vi "r3_Pick&Place_module_sensor.vi"() -> ()   [LabVIEW 2016]
uses:
  Classes/Controllers/I-O/Copy of NI-DAQ Folder/NI-DAQ.lvclass
  D:/INTT/V1/Classes/Controllers/I-O/Copy of I-O Folder/I-O.lvclass
  Classes/Controllers/Dispenser/Copy of Ultimus V2 Folder/Ultimus V2.lvclass
  <vilib>/Analysis/coordinate.llb/2D Cartesian Coordinate Rotation (Scalar).vi
  <vilib>/Utility/file.llb/Read Delimited Spreadsheet (DBL).vi
  <vilib>/Utility/file.llb/Write Delimited Spreadsheet (DBL).vi
  Classes/Controllers/Motion/Copy of Motion Folder/Motion.lvclass
  Classes/Controllers/Camera/Copy of Controller Folder/Controller.lvclass
  <vilib>/Analysis/NI_AALPro.lvlib
  Classes/Controllers/I-O/Copy of I-O Folder/I-O.lvclass
panel:
  in  "sensor pad offset":dbl[][](array[numeric])=[[0.01279, -0.02707, 0.0, 0.0], [0.00738, -0.02377, 0.0, 0.0]]
  out "Sample on HDI aspect to drawing":dbl[][](array[numeric]) format="%#_8g"
  in  "HDI sensor pad positions":dbl[][](array[numeric]) format="%#_12g"
  in  "Values":bool[](array[boolean])=[FALSE, FALSE]
  out "vacuum on?":bool[](array[boolean])
  out "Array 2":dbl[][](array[numeric])
  out "Measured PickupTool position":dbl[][](array[numeric])
  in  "sampel vacuum":i32[](array[numeric])=[15, 19]
  in  "VacChannel for sample":i32=1
  in  "TrayVaccum":bool
  in  "check height? 2":bool
  in  "check height?":bool
  out "Needle parking position":dbl[](array[numeric])
  out "GlueBox":dbl[][](array[numeric])
  out "appended array":dbl[][](array[numeric])
  in  "chip placement height compensation":dbl=-0.47 format="%#_13g"
  out "Sample on HDI":dbl[][](array[numeric]) format="%#_8g"
  in  "Sensor A/B":bool
  out "Gantry current position":dbl[](array[numeric])
  in  "READ Position":bool
  in  "Needle Height Compenstation\n(glue gap)":dbl=0.34
  in  "Needle Alignment":bool
  in  "Parking position":dbl[](array[numeric])=[500.0, 625.0, 0.0, 0.01]
  in  "GOTO":bool
  in  "Default Pickup Tool Position":dbl[][](array[numeric])=[[135.307, 678.152, 48.5457, -0.00116978], [167.269, 518.603, 48.5016, 0.000528011]]
  in  "Number of Chips/Sensors \nto be assembled":i32=1
  in  "Default HDI alignment \nmark position":dbl[](array[numeric])=[292.356, 988.848, 78.9737, -6.1789e-05]
  in  "Default HDI size":dbl[](array[numeric])=[24.3157, 231.332, -0.00999644, -6.1789e-05]
  out "# of tasks excuted":i32
  out "Chips on tray position":dbl[][](array[numeric])
  out "measured HDI size":dbl[](array[numeric])
  in  "Chip tray":dbl[](array[numeric])=[465.031, 710.639, 69.8028, 0.00407755]
  out "Sample position \non HDI":dbl[][](array[numeric]) format="%#_8g"
  in  "Inititalize":bool
  in  "Pick and place":bool
  in  "Deposit Glue":bool
  in  "Measure Pickup Tools":bool
  in  "Measure Samples on tray":bool
  out "default chip and sensor position w.r.t. 1st mark":dbl[][](array[numeric])
  in  "Assembly Type":bool
  in  "Stop":bool
  in  "Measure HDI":bool
  out "Measure HDI top-left":dbl[](array[numeric])
  # "Sensor Tray \nVacuum Channel"
  # "Chips"
  # "Sensor 0.3 -> 200 micron glue thickness\nChips 0.34-> 150 micron glue thickness"
  # "Sensors"
  # "Sensor B short"
  # "Sensors B\n(Short)"
  # "Sensors A\n(Long)"
  # "Chips : -0.47-> 60 micron height gap\n               -0.5 -> 90 micron"
  # "Sensor A long"
  # "ACTIONS"
  # "HDI infomation"
  # "sensor"
  # "chips use channel 0, 2\nsensors use channel 0, 1"
  # "sensor height 69.8471\nchip height 84.693"
  # "Pick and Place"
  # "TYPE A: \nX: 0.01279\nY: -0.02707"
  # "TYPE B: \nX: 0.00738\nY: -0.02377"
  # "type A"
  # "type B"
  # "type A"
  # "type B"
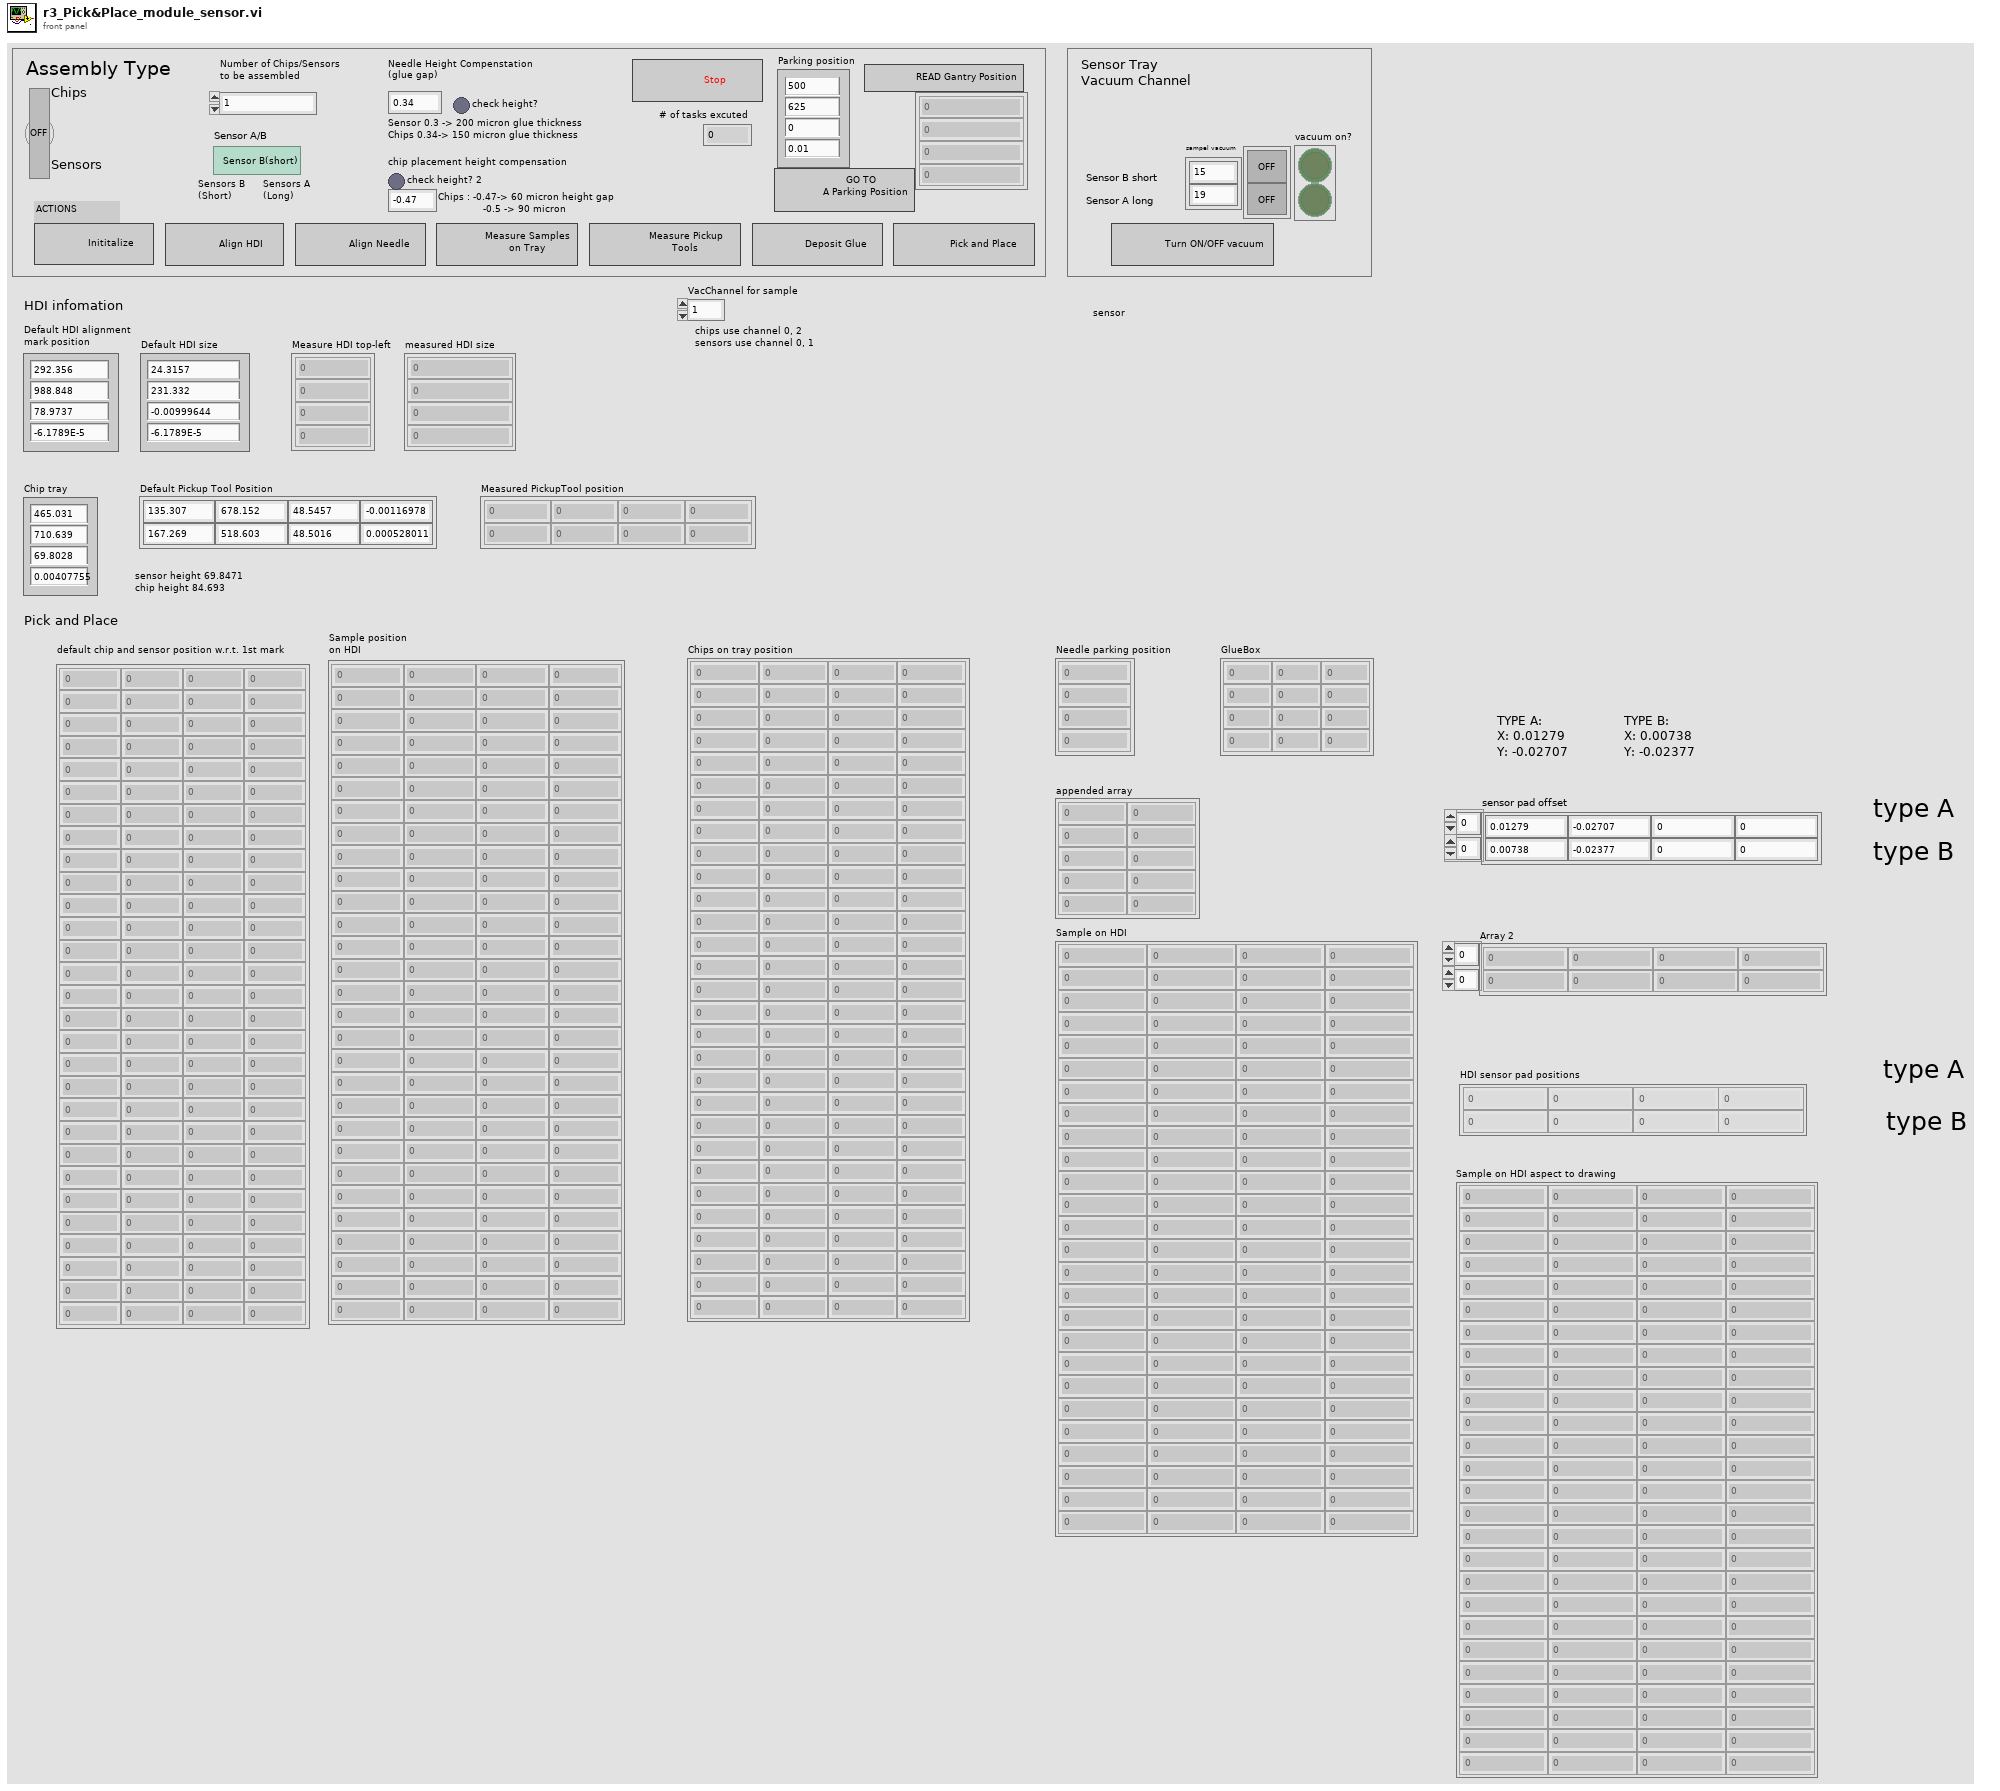
[diagram p1: front panel]
types:
  T1 = typedef "Controller.lvclass/Controllers.ctl" = cluster{"Copy of Motion.lvclass":refnum<class "Motion.lvclass">, "Copy of I-O.lvclass":refnum<class "I-O.lvclass">, "Copy of Dispenser.lvclass":refnum<class "Dispenser.lvclass">}
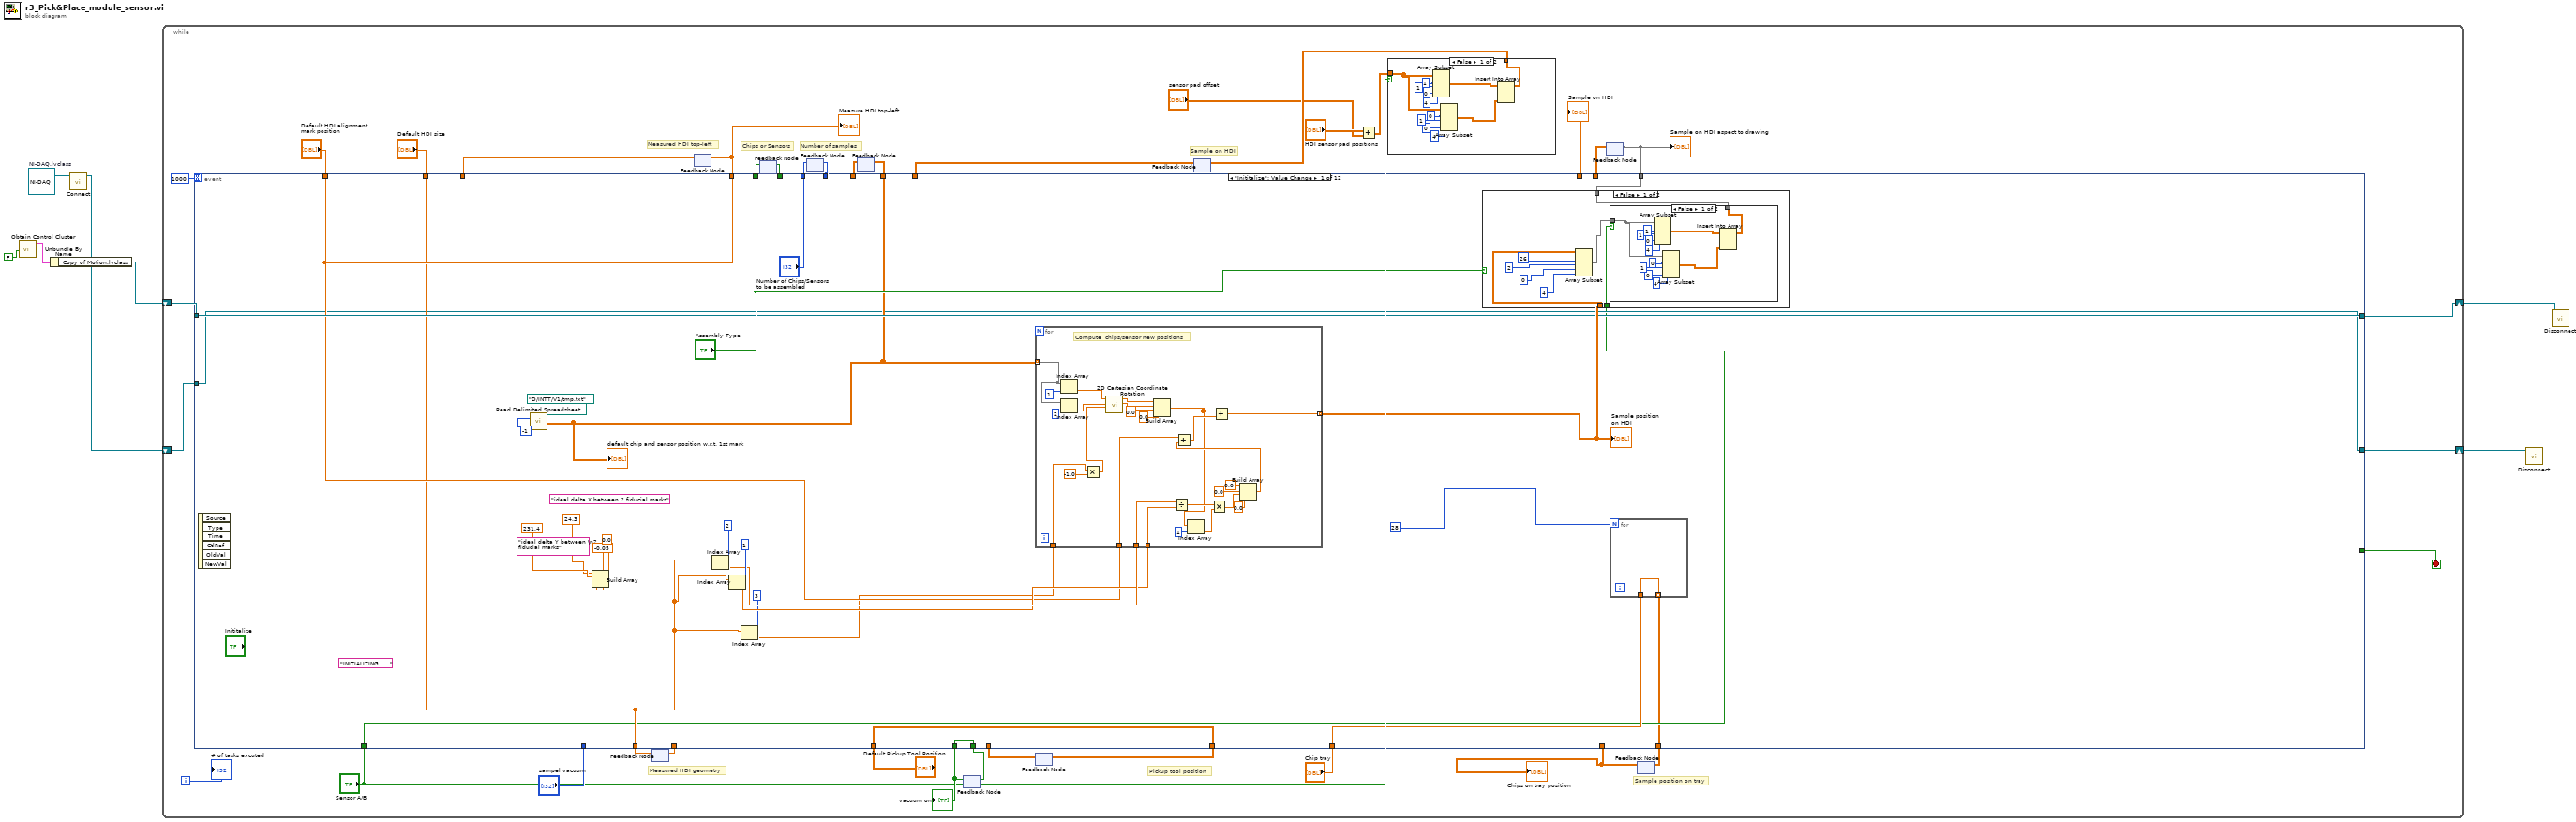
[diagram p0: block diagram]
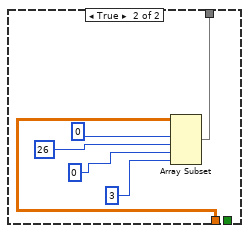
[diagram p4: hidden frame]
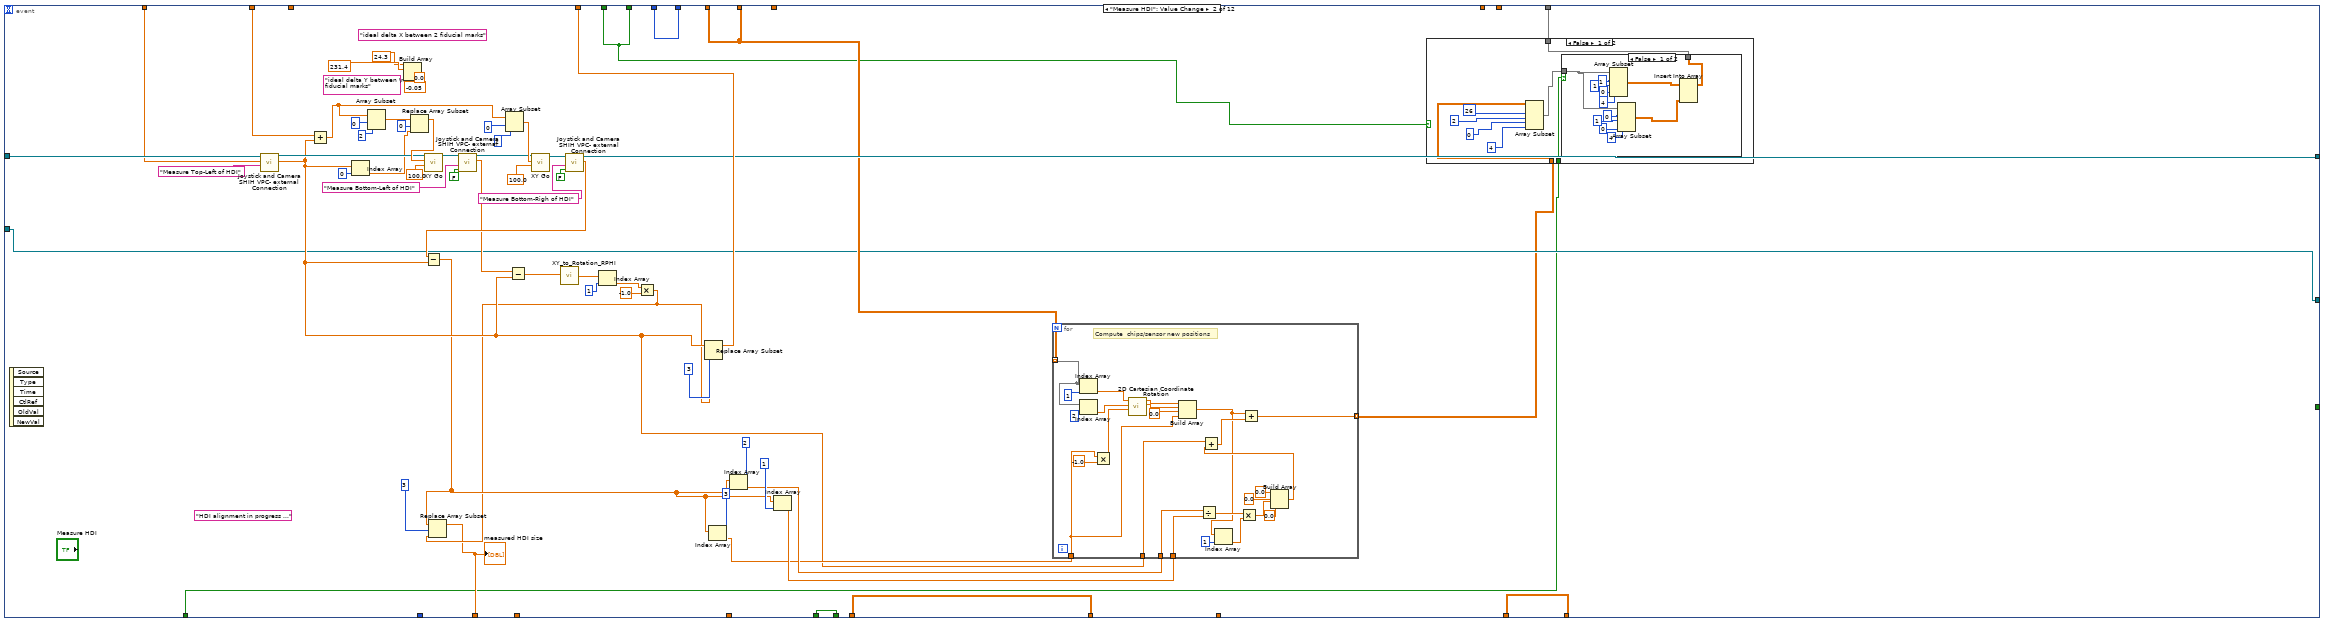
[diagram p5: hidden frame]
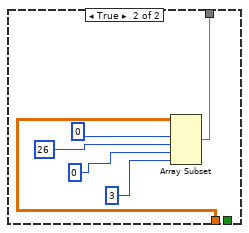
[diagram p7: hidden frame]
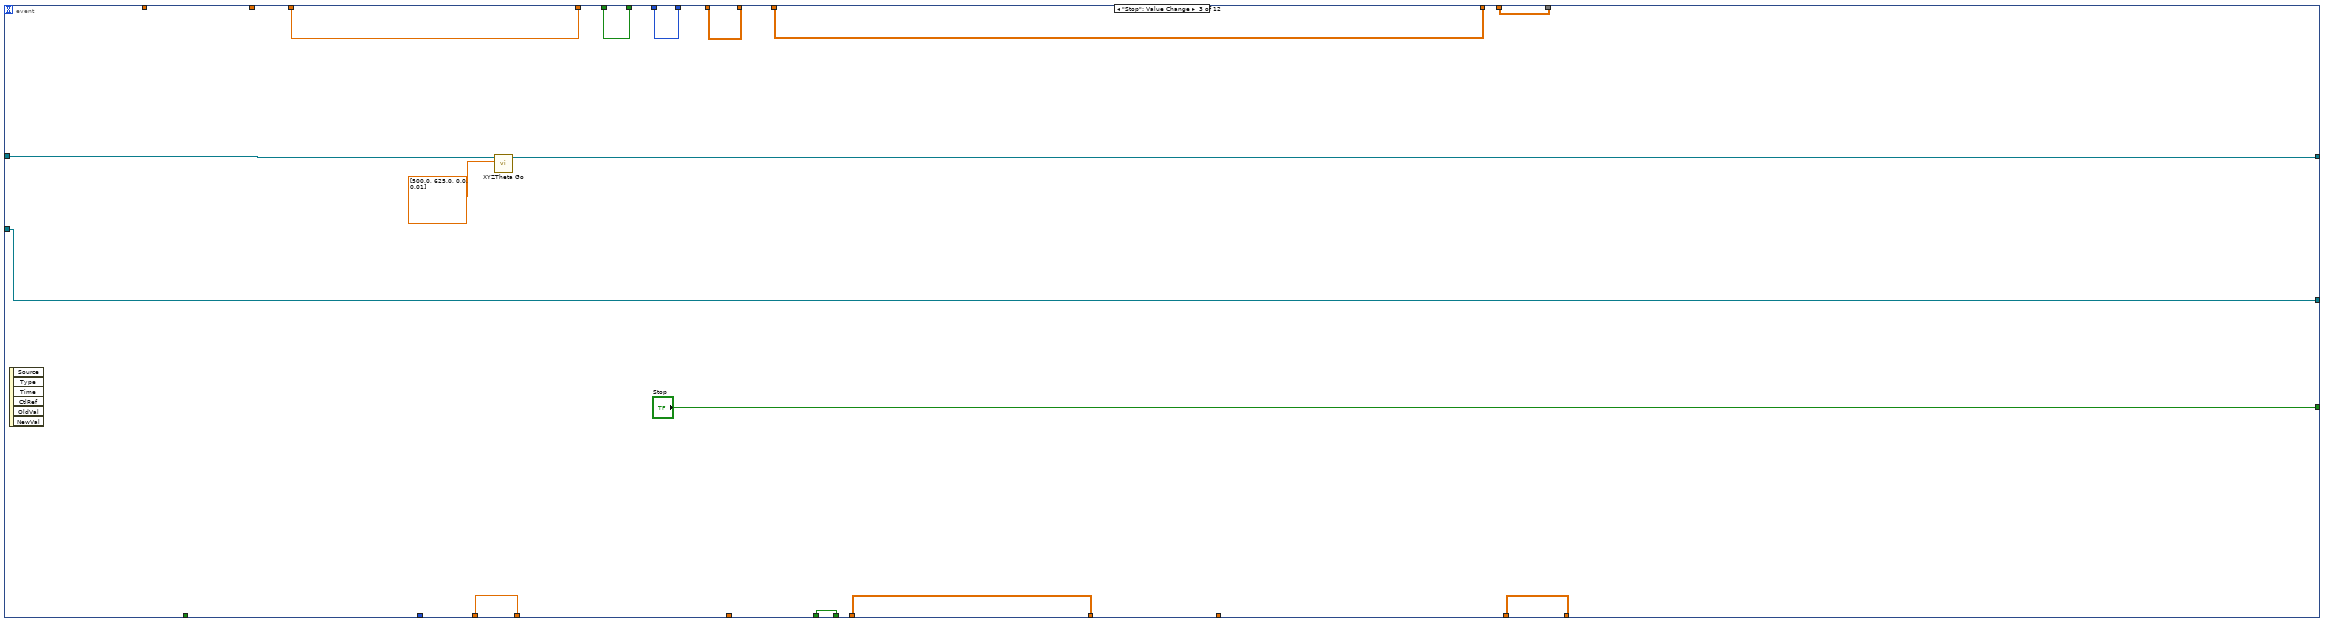
[diagram p8: hidden frame]
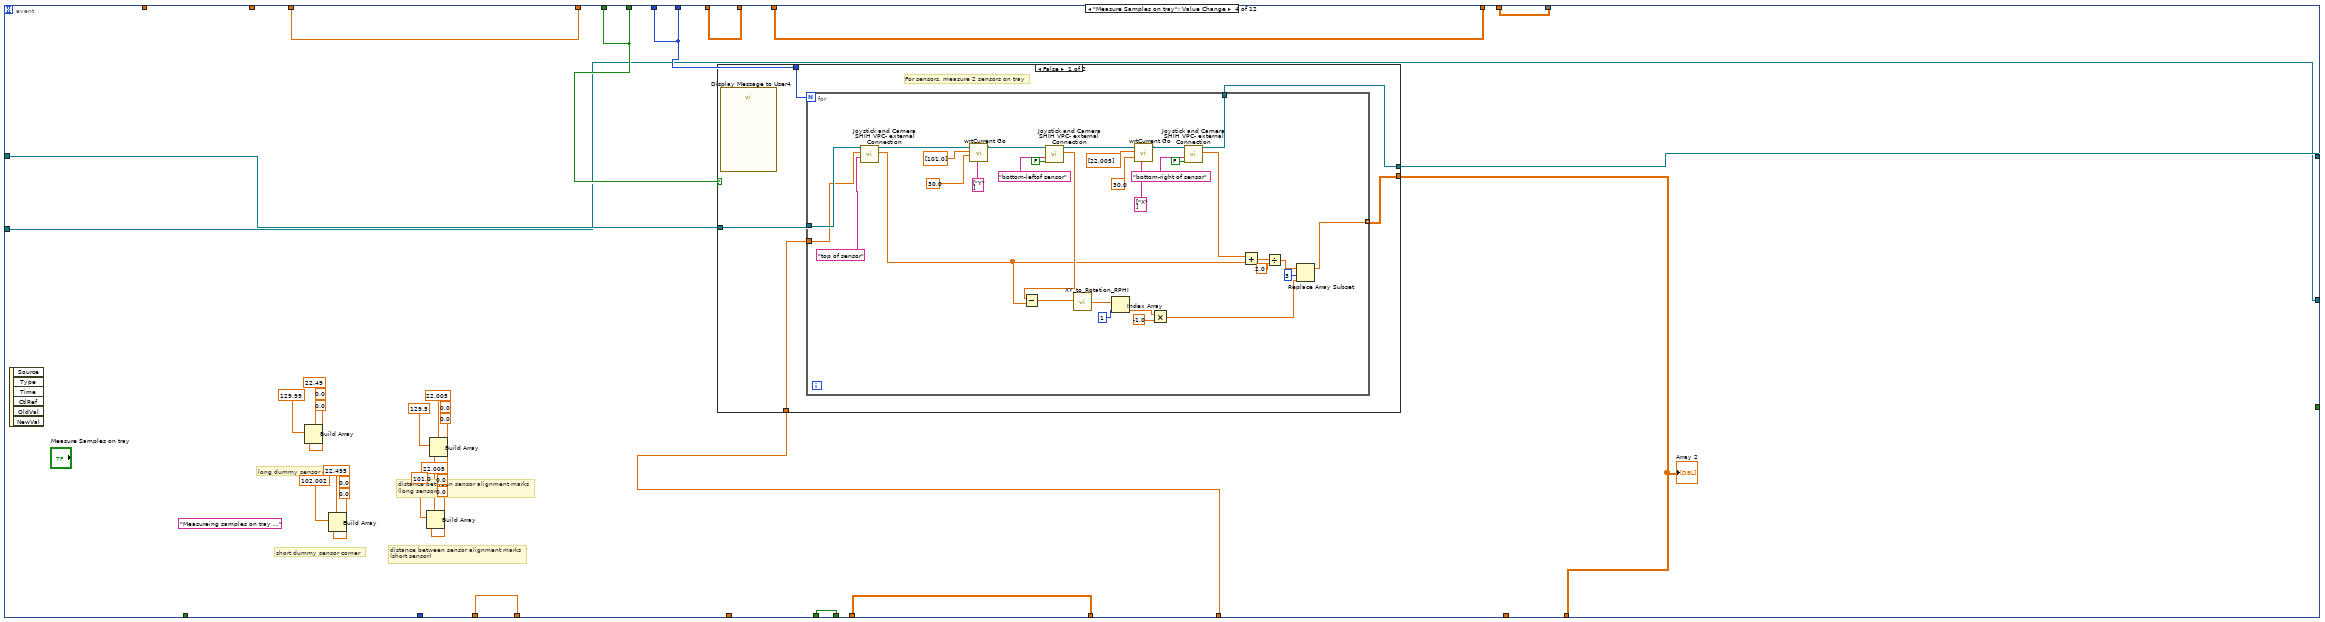
[diagram p9: hidden frame]
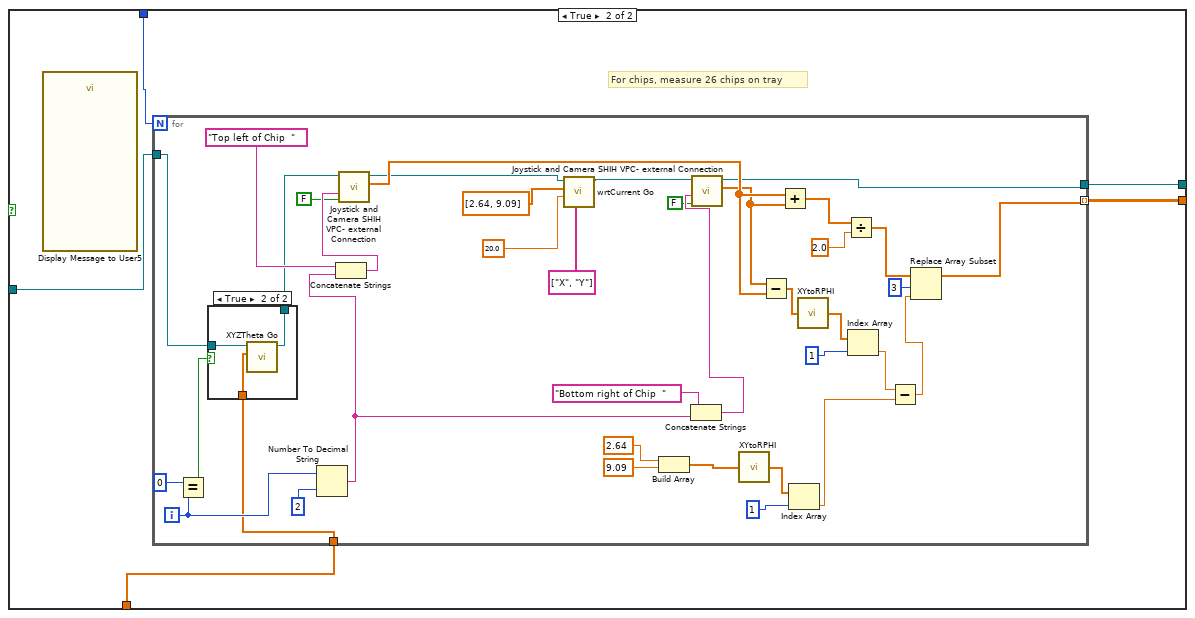
[diagram p10: hidden frame]
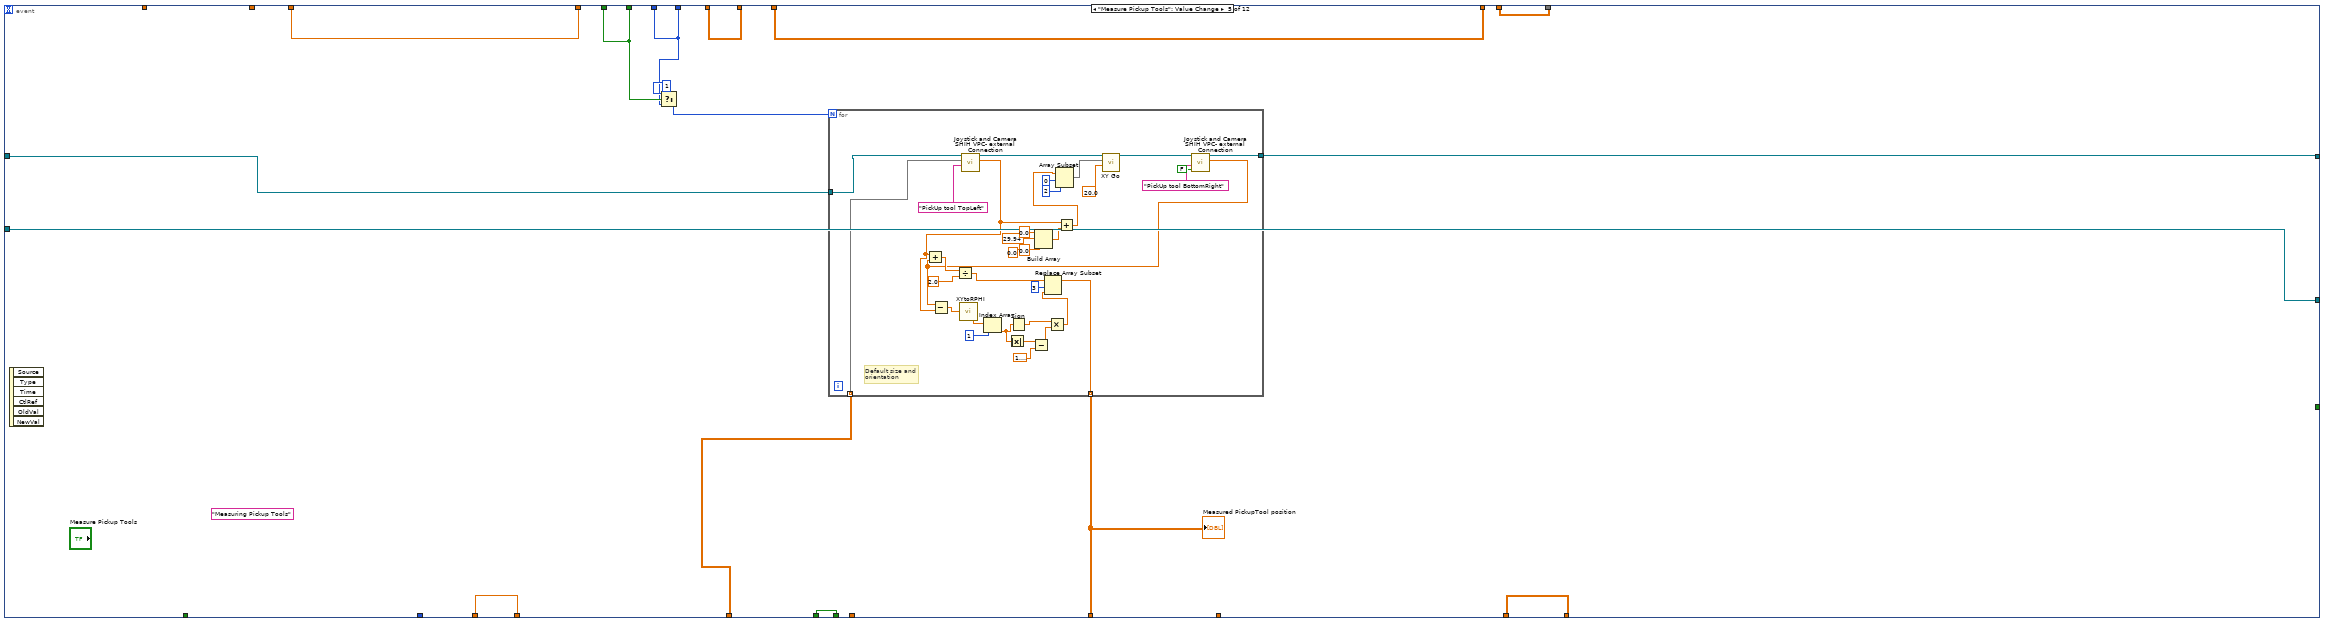
[diagram p12: hidden frame]
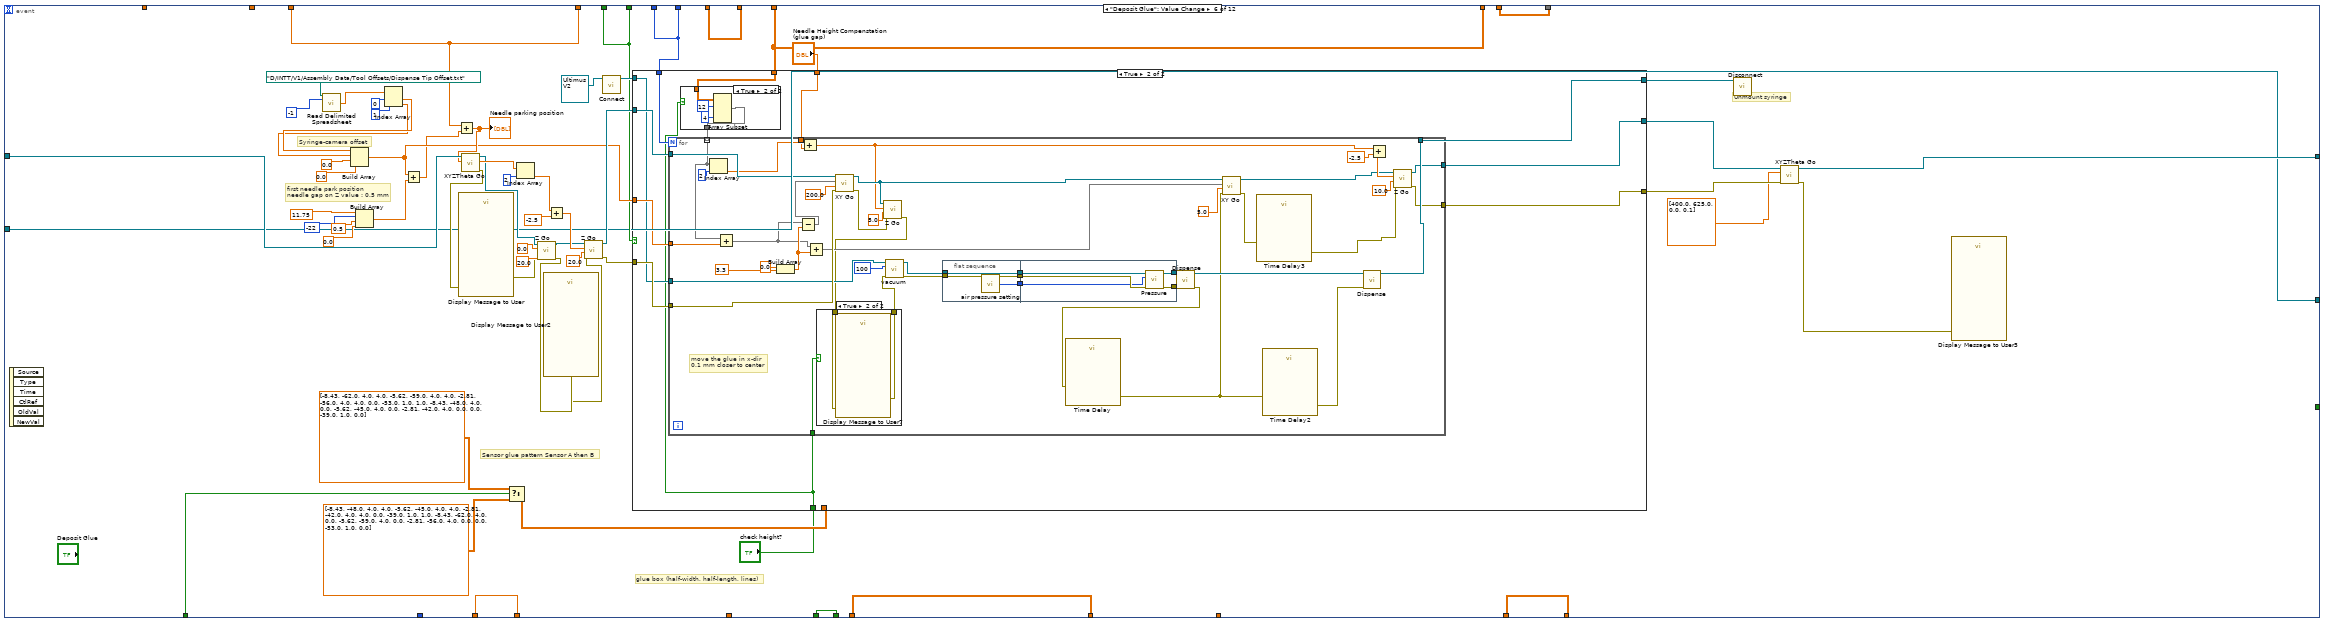
[diagram p13: hidden frame]
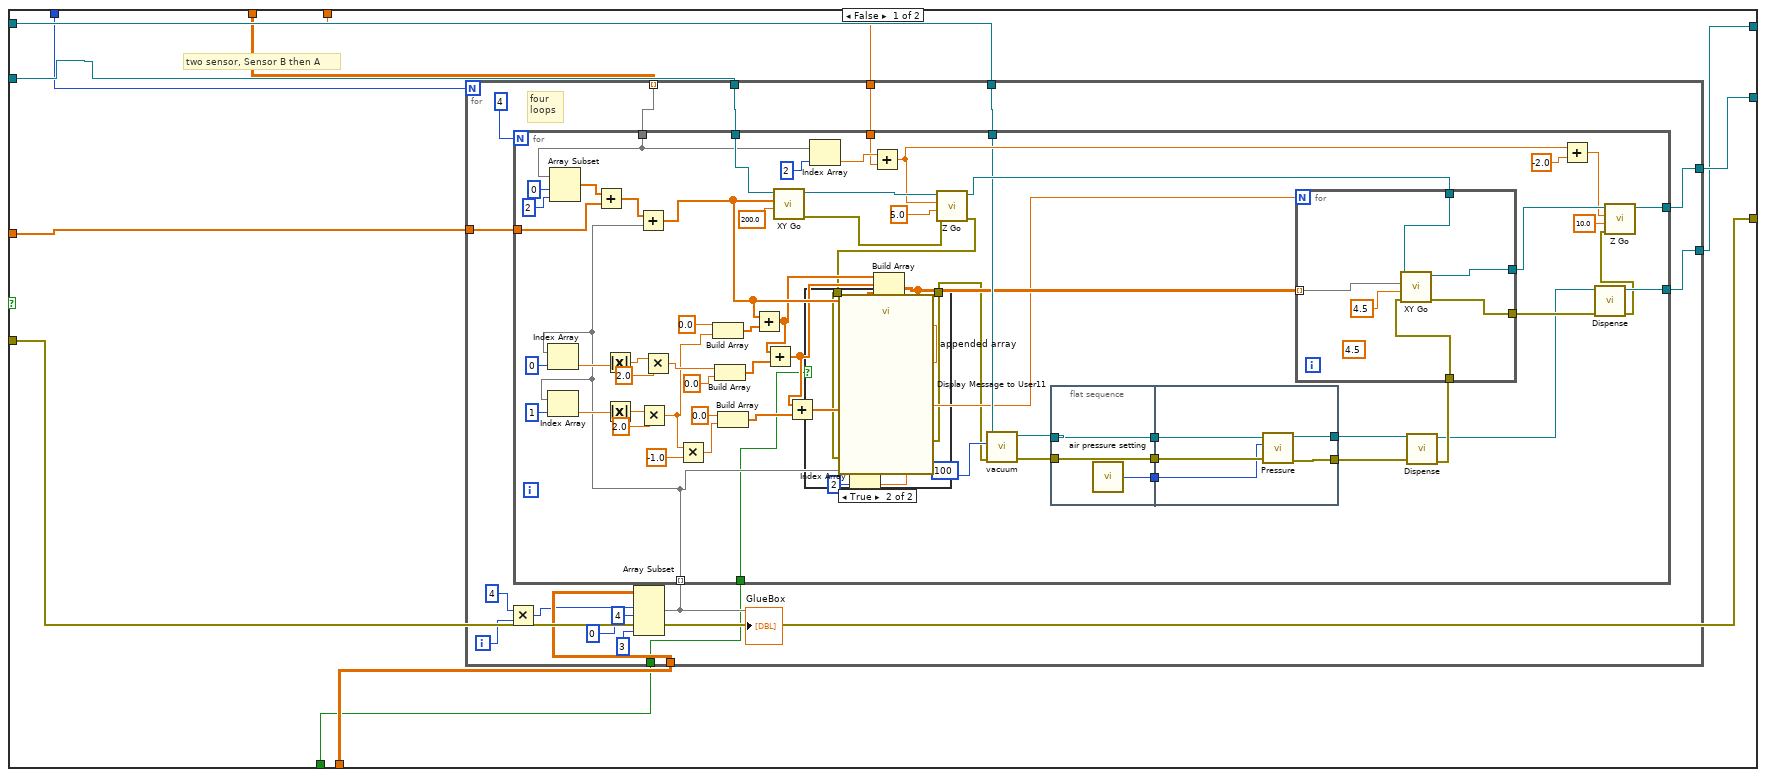
[diagram p14: hidden frame]
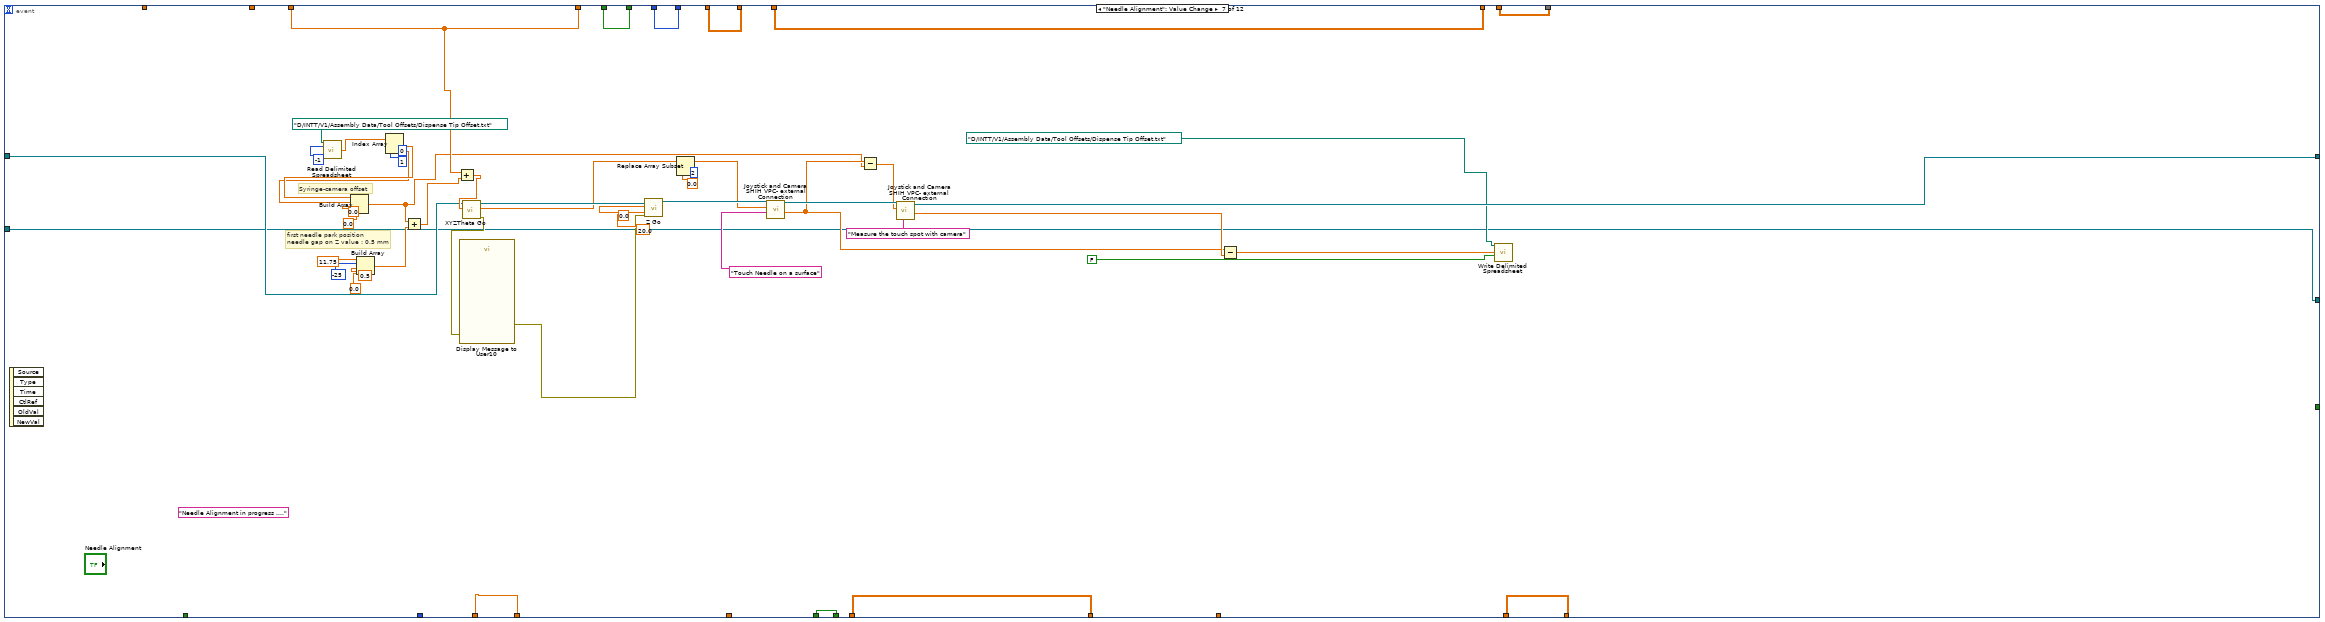
[diagram p18: hidden frame]
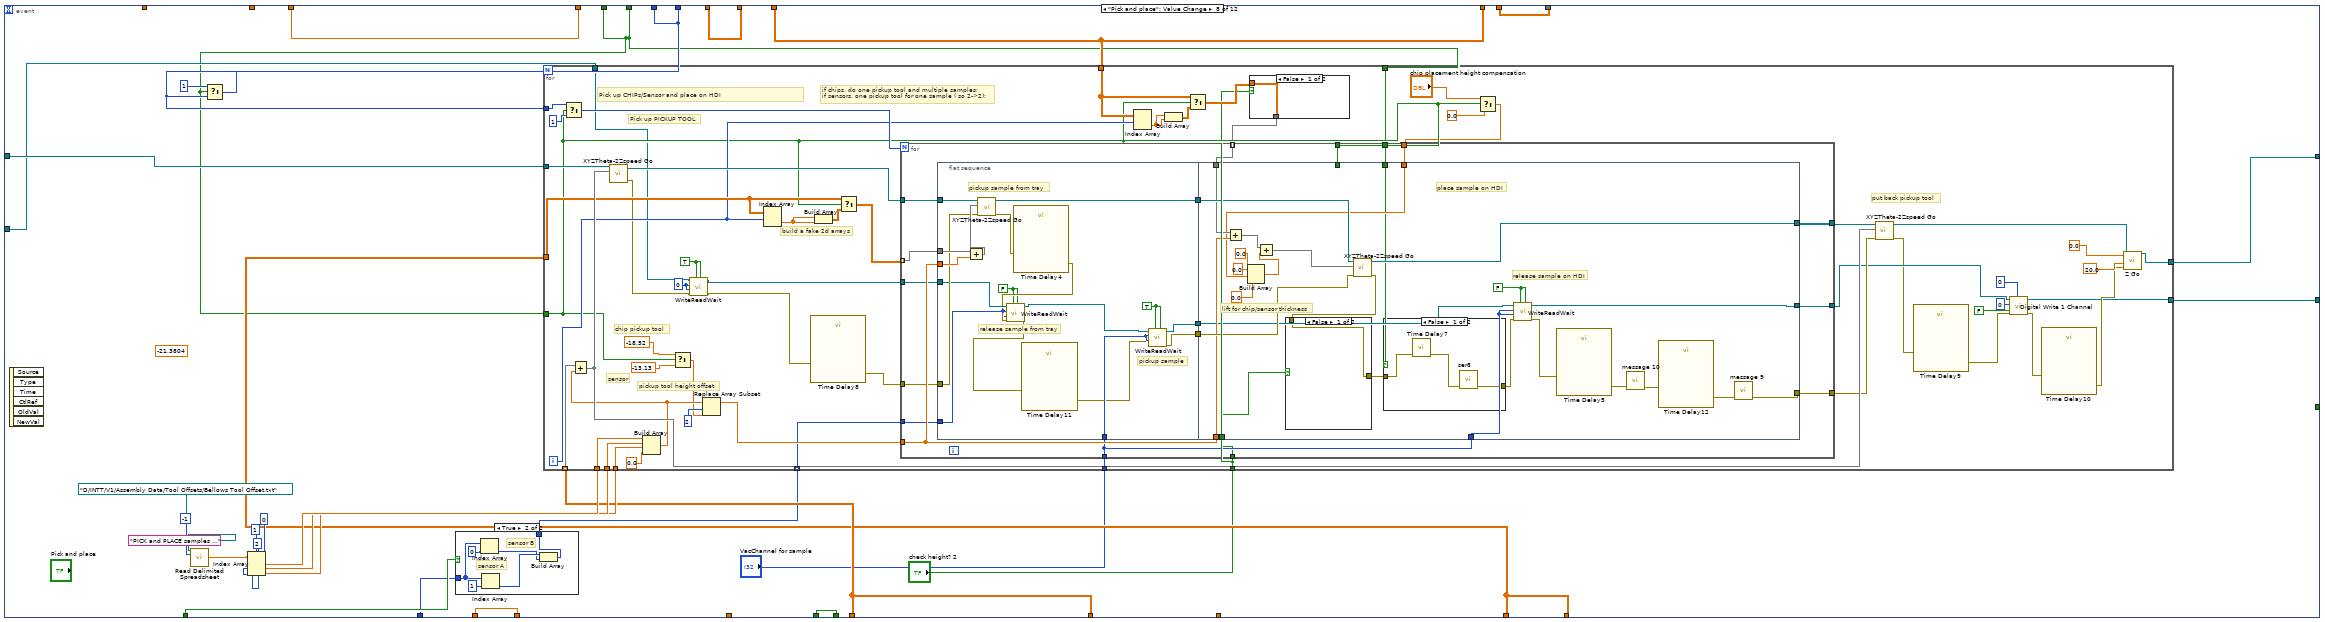
[diagram p19: hidden frame]
diagram:
  w3 = refnum<class "NI-DAQ.lvclass"> refnum  # NI-DAQ.lvclass
  n1 = call "Obtain Control Cluster.vi"("I/O"=FALSE) -> ("Control Out"=w7:T1)  [unwired: 10 in]
  n2 = Unbundle By Name(w7) -> ("Copy of Motion.lvclass"=w5:refnum<class "Motion.lvclass">)
  n3 = call-dynamic "Connect.vi"("NI-DAQ in"=w3) -> ("NI-DAQ out"=w2:refnum<class "NI-DAQ.lvclass">)  [unwired: 9 in, 1 out]
  n4 = while {
    shift-right: [w32] -> w4
    shift-left: w5 -> [w44]
    shift-right: [w20] -> w1
    shift-left: w2 -> [w21]
    i -> [w31]
    stop <- w43 stop-if-true
    # "Pickup tool position"
    # "Chips or Sensors"
    # "Number of samples"
    # "Measured HDI geometry"
    # "Sample position on tray"
    # "Measured HDI top-left"
    # "Sample on HDI"
    n5 = feedback #1() -> (w39:dbl[])  [unwired: 1 in]
    n6 = feedback #2() -> (w41:dbl[])  [unwired: 1 in]
    n7 = feedback #3() -> (w36:bool)  [unwired: 1 in]
    n8 = feedback #4() -> (w30:i32)  [unwired: 1 in]
    n9 = feedback #5() -> (w25:dbl[][])  [unwired: 1 in]
    n10 = feedback #6() -> (w17:bool[])  [unwired: 1 in]
    n11 = feedback #7() -> (w33:dbl[][])  [unwired: 1 in]
    n12 = feedback #8() -> (w38:dbl[][])  [unwired: 1 in]
    n13 = Add(x="HDI sensor pad positions", y="sensor pad offset") -> (x+y=w9:dbl[][])
    n14 = case shown="False" "Sensor A/B" {
      tunnel: w9 -> [w48 w57]
      tunnel: [w45 w57] -> w15
      frame False {
        n15 = Array Subset(array=w48, index (row)=1 ("index"), length (row)=1 ("length"), index (col)=0 ("index"), length (col)=4 ("length")) -> (w47:dbl[][])
        n16 = Array Subset(array=w48, index (row)=0 ("index"), length (row)=1 ("length"), index (col)=0 ("index"), length (col)=4 ("length")) -> (w46:dbl[][])
        n17 = Insert Into Array(array=w47, new element=w46) -> (w45:dbl[][])  [unwired: 2 in]
      }
      frame True {
      }
    }
    n18 = feedback-in #8(w15) -> ()
    n19 = feedback #9() -> (w12:dbl[][])  [unwired: 1 in]
    n20 = feedback #10() -> (w22:dbl[][])  [unwired: 1 in]
    "Chips on tray position" <- w22
    n21 = event shown="[0] \"Inititalize\": Value Change" {
      selector: _ -> [_ _ _ _ _ _ _ _ _ _ _ _]
      dyn-events: _ -> [_ _ _ _ _ _ _ _ _ _ _ _]
      timeout: 1000 -> [_ _ _ _ _ _ _ _ _ _ _ _]
      tunnel: w44 -> [w71 w198 w265 w295 w394 w463 w689 w746 w892 w915 w940 w944]
      tunnel: [_ _ "Stop" _ _ _ _ _ _ _ _ _] -> w43
      tunnel: [w68 w195 w258 w289 w385 w444 w697 w730 w901 w909 w936 w954] -> w42
      tunnel: w41 -> [_ _ w258 w289 w385 w444 w697 w730 w901 w909 w936 w954]
      tunnel: ["Assembly Type" w142 w262 w293 w390 w447 w696 w720 w900 w910 w937 w953] -> w37
      tunnel: [w64 w145 w257 w288 w384 w440 w692 w729 w896 w908 w935 w948] -> w40
      tunnel: w39 -> [_ _ w257 w288 w384 w440 w692 w729 w896 w908 w935 w948]
      tunnel: [_ _ w259 w290 w387 w446 w693 w735 w897 w913 w939 w942] -> w14
      tunnel: w38 -> [_ _ w259 w290 w387 w446 w693 w735 w897 w913 w939 w942]
      tunnel: w36 -> [_ w142 w262 w293 w390 w447 w696 w720 w900 w910 w937 w953]
      tunnel: w30 -> [_ w186 w261 w292 w389 w445 w695 w732 w899 w911 w932 w952]
      tunnel: [w58 w184 w255 w269 w383 w442 w690 w733 w894 w906 w933 w950] -> w35
      tunnel: w22 -> [_ w184 w255 _ w383 w442 w690 w733 w894 w906 w933 w950]
      tunnel: [w67 w185 w256 w287 w393 w441 w691 w734 w895 w907 w934 w949] -> w34
      tunnel: w33 -> [_ w185 w256 w287 _ w441 w691 w734 w895 w907 w934 w949]
      tunnel: [w71 w194 w263 w294 w392 w448 w681 w736 w891 w914 w940 w944] -> w32
      tunnel: ["Number of Chips/Sensors \nto be assembled" w186 w261 w292 w389 w445 w695 w732 w899 w911 w932 w952] -> w29
      tunnel: "Default HDI alignment \nmark position" -> [w68 w193 _ _ _ _ _ _ _ _ _ _]
      tunnel: "Default HDI size" -> [w64 w192 _ _ _ _ _ _ _ _ _ _]
      tunnel: [w69 w187 w260 w291 w386 w439 w694 w731 w898 w912 w938 w951] -> w26
      tunnel: w25 -> [_ w187 w260 w291 w386 w439 w694 w731 w898 w912 w938 w951]
      tunnel: "Default Pickup Tool Position" -> [w67 _ _ _ w388 _ _ _ _ _ _ _]
      tunnel: "Chip tray" -> [w66 _ _ w286 _ _ _ _ _ _ _ _]
      tunnel: "Sensor A/B" -> [w61 w139 _ _ _ w438 _ w728 _ _ _ _]
      tunnel: w21 -> [w62 w144 w253 w268 w382 w432 w672 w725 w893 w904 w931 w945]
      tunnel: [w62 w144 w253 w268 w382 w432 w672 w726 w893 w904 w917 w943] -> w20
      tunnel: "sampel vacuum" -> [_ _ _ _ _ _ _ w722 _ _ w919 w946]
      tunnel: [w60 w143 w252 w267 w381 w431 w671 w721 w889 w903 w918 w947] -> w18
      tunnel: w17 -> [w60 w143 w252 w267 w381 w431 w671 w721 w889 w903 w918 _]
      tunnel: [w59 w140 w251 w266 w380 w430 w670 w719 w888 w902 w916 w941] -> w13
      tunnel: w12 -> [_ _ w251 w266 w380 w430 w670 w719 w888 w902 w916 w941]
      event "Inititalize": Value Change {
        (unwired) "INITIALIZING ....." ("String")
        (unwired) "ideal delta Y between \n2 fiducial marks"
        (unwired) "ideal delta X between 2 fiducial marks"
        n22 = event-data() -> ()  [unwired: 1 in, 6 out]
        n23 = call-poly <vilib>:"Read Delimited Spreadsheet.vi"("file path (dialog if empty)"=path "D:/INTT/V1/tmp.txt", "number of rows (all:-1)"=-1) -> ("all rows"=w69:dbl[][])  [unwired: 8 in, 5 out]
        "default chip and sensor position w.r.t. 1st mark" <- w69
        n24 = Build Array(24.3 ("y"), 231.4 ("y"), 0.0 ("element"), -0.05 ("element")) -> ()  [unwired: 1 out]
        n25 = Index Array(array=w64, index=2) -> (element=w80:dbl)
        n26 = Index Array(array=w64, index=1) -> (element=w79:dbl)
        n27 = Index Array(array=w64, index=3) -> (element=w63:dbl)
        n28 = for {
          tunnel: w69 -> [w131] mode=indexing
          tunnel: w63 -> [w114]
          tunnel: w68 -> [w123]
          tunnel: [w130] -> w73 mode=indexing
          tunnel: w80 -> [w129]
          tunnel: w79 -> [w120]
          # "Compute  chips/sensor new positions"
          n29 = Index Array(array=w131, index=1) -> (element=w135:dbl)
          n30 = Index Array(array=w131, index=2) -> (element=w134:dbl)
          n31 = Multiply(x=w114, y=-1.0) -> (x*y=w115:dbl)
          n32 = call-poly <vilib>:"2D Cartesian Coordinate Rotation.vi"("theta"=w115, "y"=w134, "x"=w135) -> ("y out"=w137:dbl, "x out"=w136:dbl)  [unwired: 6 in, 1 out]
          n33 = Build Array(w136, w137, 0.0 ("element"), 0.0 ("element")) -> (w117:dbl[])
          n34 = Divide(x=w129, y=w120) -> (x/y=w128:dbl)
          n35 = Index Array(array=w117, index=1) -> (element=w118:dbl)
          n36 = Multiply(x=w128, y=w118) -> (x*y=w124:dbl)
          n37 = Build Array(0.0 ("element"), 0.0 ("element"), w124, 0.0 ("element")) -> (w122:dbl[])
          n38 = Add(x=w123, y=w122) -> (x+y=w121:dbl[])
          n39 = Add(x=w117, y=w121) -> (x+y=w130:dbl[])
        }
        "Sample position \non HDI" <- w73
        n40 = case shown="False" "Assembly Type" {
          tunnel: w73 -> [w88 w108]
          tunnel: [w86 w106] -> w59
          tunnel: w61 -> [w85 _]
          frame False {
            n41 = Array Subset(array=w88, index (row)=26 ("index"), length (row)=2 ("length"), index (col)=0, length (col)=4 ("length")) -> (w87:dbl[][])
            n42 = case shown="False" w85 {
              tunnel: w87 -> [w96 w105]
              tunnel: [w93 w105] -> w86
              frame False {
                n43 = Array Subset(array=w96, index (row)=1 ("index"), length (row)=1 ("length"), index (col)=0 ("index"), length (col)=4 ("length")) -> (w95:dbl[][])
                n44 = Array Subset(array=w96, index (row)=0 ("index"), length (row)=1 ("length"), index (col)=0 ("index"), length (col)=4 ("length")) -> (w94:dbl[][])
                n45 = Insert Into Array(array=w95, new element=w94) -> (w93:dbl[][])  [unwired: 2 in]
              }
              frame True {
              }
            }
          }
          frame True {
            n46 = Array Subset(array=w108, index (row)=0 ("index"), length (row)=26 ("length"), index (col)=0, length (col)=3 ("length")) -> (w106:dbl[][])
          }
        }
        n47 = for {
          N: 28 -> [_]
          tunnel: w66 -> [w112]
          tunnel: [w112] -> w58 mode=indexing
        }
      }
      event "Measure HDI": Value Change {
        (unwired) "ideal delta Y between \n2 fiducial marks"
        (unwired) "ideal delta X between 2 fiducial marks"
        (unwired) "HDI alignment in progress ..." ("String")
        n48 = event-data() -> ()  [unwired: 1 in, 6 out]
        n49 = call "Joystick and Camera SHIH VPC- external Connection.vi"("Motion in"=w198, "XYZTheta"=w193, "Measurement Point"="Measure Top-Left of HDI") -> ("Motion out"=w162:refnum<class "Motion.lvclass">, "Sum"=w151:dbl[])  [unwired: 4 in, 2 out]
        n50 = Add(x=w192, y=w151) -> (x+y=w166:dbl[])
        n51 = Index Array(array=w151, index=0) -> (element=w153:dbl)
        n52 = Array Subset(array=w166, index=0, length=2) -> (w165:dbl[])
        n53 = Build Array(24.3 ("y"), 231.4 ("y"), 0.0 ("element"), -0.05 ("element")) -> ()  [unwired: 1 out]
        n54 = Replace Array Subset(array=w165, new element=w153, index=0) -> (w163:dbl[])
        n55 = call-dynamic "XY Go.vi"("Speed"=100.0, "XY"=w163, "Motion in"=w162) -> ("Motion out"=w170:refnum<class "Motion.lvclass">)  [unwired: 7 in, 1 out]
        n56 = call "Joystick and Camera SHIH VPC- external Connection.vi"("Motion in"=w170, "Measurement Point"="Measure Bottom-Left of HDI", "Inital GO"=FALSE) -> ("Motion out"=w161:refnum<class "Motion.lvclass">, "Sum"=w152:dbl[])  [unwired: 4 in, 2 out]
        n57 = Array Subset(array=w166, index=0, length=2) -> (w176:dbl[])
        n58 = Subtract(x=w152, y=w151) -> (x-y=w160:dbl[])
        n59 = call-dynamic "XY Go.vi"("Speed"=100.0, "XY"=w176, "Motion in"=w161) -> ("Motion out"=w180:refnum<class "Motion.lvclass">)  [unwired: 7 in, 1 out]
        n60 = call "XY_to_Rotation_RPHI.vi"("X-Y"=w160) -> ("r-phi"=w156:dbl[])
        n61 = call "Joystick and Camera SHIH VPC- external Connection.vi"("Motion in"=w180, "Measurement Point"="Measure Bottom-Righ of HDI", "Inital GO"=FALSE) -> ("Motion out"=w194:refnum<class "Motion.lvclass">, "Sum"=w197:dbl[])  [unwired: 4 in, 2 out]
        n62 = Subtract(x=w197, y=w151) -> (x-y=w148:dbl[])
        n63 = Index Array(array=w156, index=1) -> (element=w149:dbl)
        n64 = Multiply(x=w149, y=-1.0) -> (x*y=w146:dbl)
        n65 = Replace Array Subset(array=w148, new element=w146, index=3) -> (w145:dbl[])
        "measured HDI size" <- w145
        n66 = Replace Array Subset(array=w151, new element=w146, index=3) -> (w195:dbl[])
        n67 = Index Array(array=w148, index=3) -> (element=w182:dbl)
        n68 = Index Array(array=w148, index=2) -> (element=w189:dbl)
        n69 = Index Array(array=w148, index=1) -> (element=w188:dbl)
        n70 = for {
          tunnel: w187 -> [w243] mode=indexing
          tunnel: w182 -> [w227]
          tunnel: w151 -> [w235]
          tunnel: [w242] -> w141 mode=indexing
          tunnel: w189 -> [w241]
          tunnel: w188 -> [w232]
          # "Compute  chips/sensor new positions"
          n71 = Index Array(array=w243, index=1) -> (element=w247:dbl)
          n72 = Index Array(array=w243, index=2) -> (element=w246:dbl)
          n73 = Multiply(x=w227, y=-1.0) -> (x*y=w226:dbl)
          n74 = call-poly <vilib>:"2D Cartesian Coordinate Rotation.vi"("theta"=w226, "y"=w246, "x"=w247) -> ("y out"=w249:dbl, "x out"=w248:dbl)  [unwired: 6 in, 1 out]
          n75 = Build Array(w248, w249, 0.0 ("element"), w227) -> (w229:dbl[])
          n76 = Divide(x=w241, y=w232) -> (x/y=w240:dbl)
          n77 = Index Array(array=w229, index=1) -> (element=w230:dbl)
          n78 = Multiply(x=w240, y=w230) -> (x*y=w236:dbl)
          n79 = Build Array(0.0 ("element"), 0.0 ("element"), w236, 0.0 ("element")) -> (w234:dbl[])
          n80 = Add(x=w235, y=w234) -> (x+y=w233:dbl[])
          n81 = Add(x=w229, y=w233) -> (x+y=w242:dbl[])
        }
        n82 = case shown="False" w142 {
          tunnel: w141 -> [w202 w222]
          tunnel: [w200 w220] -> w140
          tunnel: w139 -> [w199 _]
          frame False {
            n83 = Array Subset(array=w202, index (row)=26 ("index"), length (row)=2 ("length"), index (col)=0, length (col)=4 ("length")) -> (w201:dbl[][])
            n84 = case shown="False" w199 {
              tunnel: w201 -> [w210 w219]
              tunnel: [w207 w219] -> w200
              frame False {
                n85 = Array Subset(array=w210, index (row)=1 ("index"), length (row)=1 ("length"), index (col)=0 ("index"), length (col)=4 ("length")) -> (w209:dbl[][])
                n86 = Array Subset(array=w210, index (row)=0 ("index"), length (row)=1 ("length"), index (col)=0 ("index"), length (col)=4 ("length")) -> (w208:dbl[][])
                n87 = Insert Into Array(array=w209, new element=w208) -> (w207:dbl[][])  [unwired: 2 in]
              }
              frame True {
              }
            }
          }
          frame True {
            n88 = Array Subset(array=w222, index (row)=0 ("index"), length (row)=26 ("length"), index (col)=0, length (col)=3 ("length")) -> (w220:dbl[][])
          }
        }
      }
      event "Stop": Value Change {
        n89 = event-data() -> ()  [unwired: 1 in, 6 out]
        n90 = call "XYZTheta Go.vi"("XYZTheta In"=dbl[] [500.0, 625.0, 0.0, 0.01], "Motion in"=w265) -> ("Motion out"=w263:refnum<class "Motion.lvclass">)  [unwired: 7 in, 2 out]
      }
      event "Measure Samples on tray": Value Change {
        (unwired) "Measureing samples on tray ..." ("String")
        # "long dummy sensor corner"
        # "short dummy sensor corner"
        # "distance between sensor alignment marks\n(short sensor)"
        # "distance between sensor alignment marks\n(long sensor)"
        n91 = event-data() -> ()  [unwired: 1 in, 6 out]
        n92 = Build Array(22.49 ("element"), 129.99 ("element"), 0.0 ("element"), 0.0 ("element")) -> ()  [unwired: 1 out]
        n93 = Build Array(22.495 ("element"), 102.002 ("element"), 0.0 ("element"), 0.0 ("element")) -> ()  [unwired: 1 out]
        n94 = Build Array(22.005 ("element"), 101.0 ("element"), 0.0 ("element"), 0.0 ("element")) -> ()  [unwired: 1 out]
        n95 = Build Array(22.005 ("element"), 129.5 ("element"), 0.0 ("element"), 0.0 ("element")) -> ()  [unwired: 1 out]
        n96 = case shown="False" w293 {
          tunnel: [w297 w337] -> w269
          tunnel: w295 -> [w300 w336]
          tunnel: [w296 w335] -> w294
          tunnel: w292 -> [w299 w334]
          tunnel: w286 -> [w298 w333]
          frame False {
            # "For sensors, measure 2 sensors on tray"
            n97 = call "Display Message to User4"() -> ()  [unwired: 10 in, 2 out]
            n98 = for {
              N: w299 -> [_]
              tunnel: w300 -> [w332]
              tunnel: [w329] -> w296
              tunnel: [w323] -> w297 mode=indexing
              tunnel: w298 -> [w322]
              n99 = call "Joystick and Camera SHIH VPC- external Connection.vi"("Motion in"=w332, "XYZTheta"=w322, "Measurement Point"="top of sensor") -> ("Motion out"=w304:refnum<class "Motion.lvclass">, "Sum"=w311:dbl[])  [unwired: 4 in, 2 out]
              n100 = call-dynamic "wrtCurrent Go.vi"("axis names"=string[] ["Y"], "Speed"=30.0, "distances"=dbl[] [101.0], "Motion in"=w304) -> ("Motion out"=w303:refnum<class "Motion.lvclass">)  [unwired: 6 in, 1 out]
              n101 = call "Joystick and Camera SHIH VPC- external Connection.vi"("Motion in"=w303, "Measurement Point"="bottom-leftof sensor", "Inital GO"=FALSE) -> ("Motion out"=w309:refnum<class "Motion.lvclass">, "Sum"=w313:dbl[])  [unwired: 4 in, 2 out]
              n102 = Subtract(x=w313, y=w311) -> (x-y=w318:dbl[])
              n103 = call "XY_to_Rotation_RPHI.vi"("X-Y"=w318) -> ("r-phi"=w317:dbl[])
              n104 = Index Array(array=w317, index=1) -> (element=w314:dbl)
              n105 = call-dynamic "wrtCurrent Go.vi"("axis names"=string[] ["X"], "Speed"=30.0, "distances"=dbl[] [22.005], "Motion in"=w309) -> ("Motion out"=w310:refnum<class "Motion.lvclass">)  [unwired: 6 in, 1 out]
              n106 = Multiply(x=w314, y=-1.0) -> (x*y=w312:dbl)
              n107 = call "Joystick and Camera SHIH VPC- external Connection.vi"("Motion in"=w310, "Measurement Point"="bottom-right of sensor", "Inital GO"=FALSE) -> ("Motion out"=w329:refnum<class "Motion.lvclass">, "Sum"=w326:dbl[])  [unwired: 4 in, 2 out]
              n108 = Add(x=w326, y=w311) -> (x+y=w327:dbl[])
              n109 = Divide(x=w327, y=2.0) -> (x/y=w325:dbl[])
              n110 = Replace Array Subset(array=w325, new element=w312, index=3) -> (w323:dbl[])
            }
          }
          frame True {
            # "For chips, measure 26 chips on tray"
            n111 = call "Display Message to User5"() -> ()  [unwired: 10 in, 2 out]
            n112 = for {
              N: w334 -> [_]
              tunnel: [w364] -> w337 mode=indexing
              tunnel: w336 -> [w348]
              tunnel: [w344] -> w335
              tunnel: w333 -> [w349]
              i -> [w352]
              n113 = Equal?(x=0, y=w352) -> (x = y?=w350:bool)
              n114 = case shown="True" w350 {
                tunnel: w349 -> [_ w379]
                tunnel: w348 -> [w376 w378]
                tunnel: [w376 w377] -> w347
                frame False {
                }
                frame True {
                  n115 = call "XYZTheta Go.vi"("XYZTheta In"=w379, "Motion in"=w378) -> ("Motion out"=w377:refnum<class "Motion.lvclass">)  [unwired: 7 in, 2 out]
                }
              }
              n116 = Number To Decimal String(number=w352, width (-)=i16 2) -> (decimal integer string=w368:string)
              n117 = Concatenate Strings("Top left of Chip  " ("string"), w368) -> (w362:string)
              n118 = call "Joystick and Camera SHIH VPC- external Connection.vi"("Motion in"=w347, "Measurement Point"=w362, "Inital GO"=FALSE) -> ("Motion out"=w341:refnum<class "Motion.lvclass">, "Sum"=w367:dbl[])  [unwired: 4 in, 2 out]
              n119 = call-dynamic "wrtCurrent Go.vi"("axis names"=string[] ["X", "Y"], "Speed"=20.0, "distances"=dbl[] [2.64, 9.09], "Motion in"=w341) -> ("Motion out"=w342:refnum<class "Motion.lvclass">)  [unwired: 6 in, 1 out]
              n120 = Build Array(2.64 ("element"), 9.09 ("element")) -> (w357:dbl[])
              n121 = Concatenate Strings("Bottom right of Chip  " ("string"), w368) -> (w346:string)
              n122 = call "Joystick and Camera SHIH VPC- external Connection.vi"("Motion in"=w342, "Measurement Point"=w346, "Inital GO"=FALSE) -> ("Motion out"=w344:refnum<class "Motion.lvclass">, "Sum"=w343:dbl[])  [unwired: 4 in, 2 out]
              n123 = call "XYtoRPHI.vi"("X-Y"=w357) -> ("r-phi"=w359:dbl[])
              n124 = Subtract(x=w343, y=w367) -> (x-y=w360:dbl[])
              n125 = Add(x=w367, y=w343) -> (x+y=w372:dbl[])
              n126 = Index Array(array=w359, index=1) -> (element=w354:dbl)
              n127 = call "XYtoRPHI.vi"("X-Y"=w360) -> ("r-phi"=w371:dbl[])
              n128 = Divide(x=w372, y=2.0) -> (x/y=w366:dbl[])
              n129 = Index Array(array=w371, index=1) -> (element=w355:dbl)
              n130 = Subtract(x=w355, y=w354) -> (x-y=w356:dbl)
              n131 = Replace Array Subset(array=w366, new element=w356, index=3) -> (w364:dbl[])
            }
          }
        }
        "Array 2" <- w269
      }
      event "Measure Pickup Tools": Value Change {
        (unwired) "Measuring Pickup Tools" ("String")
        n132 = event-data() -> ()  [unwired: 1 in, 6 out]
        n133 = Select(t=i8 1, s=w390, f=w389) -> (s? t:f=w391:i32)
        n134 = for {
          N: w391 -> [_]
          tunnel: [w419] -> w393 mode=indexing
          tunnel: w394 -> [w423]
          tunnel: [w405] -> w392
          tunnel: w388 -> [w404] mode=indexing
          # "Default size and\norientation"
          n135 = call "Joystick and Camera SHIH VPC- external Connection.vi"("Motion in"=w423, "XYZTheta"=w404, "Measurement Point"="PickUp tool TopLeft") -> ("Motion out"=w399:refnum<class "Motion.lvclass">, "Sum"=w422:dbl[])  [unwired: 4 in, 2 out]
          n136 = Build Array(0.0 ("element"), 29.94 ("element"), 0.0 ("element"), 0.0 ("element")) -> (w410:dbl[])
          n137 = Add(x=w422, y=w410) -> (x+y=w396:dbl[])
          n138 = Array Subset(array=w396, index=0, length=2) -> (w397:dbl[])
          n139 = call-dynamic "XY Go.vi"("Speed"=20.0, "XY"=w397, "Motion in"=w399) -> ("Motion out"=w398:refnum<class "Motion.lvclass">)  [unwired: 7 in, 1 out]
          n140 = call "Joystick and Camera SHIH VPC- external Connection.vi"("Motion in"=w398, "Measurement Point"="PickUp tool BottomRight", "Inital GO"=FALSE) -> ("Motion out"=w405:refnum<class "Motion.lvclass">, "Sum"=w421:dbl[])  [unwired: 4 in, 2 out]
          n141 = Add(x=w422, y=w421) -> (x+y=w428:dbl[])
          n142 = Subtract(x=w421, y=w422) -> (x-y=w420:dbl[])
          n143 = Divide(x=w428, y=2.0) -> (x/y=w425:dbl[])
          n144 = call "XYtoRPHI.vi"("X-Y"=w420) -> ("r-phi"=w426:dbl[])
          n145 = Index Array(array=w426, index=1) -> (element=w414:dbl)
          n146 = Absolute Value(x=w414) -> (abs(x)=w417:dbl)
          n147 = Sign(1:w414) -> (0:w415:dbl)
          n148 = Subtract(x=w417, y=1.5707963267948966) -> (x-y=w416:dbl)
          n149 = Multiply(x=w415, y=w416) -> (x*y=w413:dbl)
          n150 = Replace Array Subset(array=w425, new element=w413, index=3) -> (w419:dbl[])
        }
        "Measured PickupTool position" <- w393
      }
      event "Deposit Glue": Value Change {
        # "glue box (half-width, half-length, lines)"
        # "Sensor glue pattern Sensor A then B"
        # "Unmount syringe"
        # "first needle park position\nneedle gap on Z value : 0.5 mm"
        # "Syringe-camera offset"
        n151 = event-data() -> ()  [unwired: 1 in, 6 out]
        n152 = call-poly <vilib>:"Read Delimited Spreadsheet.vi"("file path (dialog if empty)"=path "D:/INTT/V1/Assembly Data/Tool Offsets/Dispense Tip Offset.txt", "number of rows (all:-1)"=-1) -> ("first row"=w483:dbl[])  [unwired: 8 in, 5 out]
        n153 = Build Array(11.75, -22, 0.5 ("element"), 0.0 ("element")) -> (w476:dbl[])
        n154 = Index Array(array=w483, index #1=0 ("index"), index #2=1 ("index")) -> (element #1=w478:dbl, element #2=w475:dbl)
        n155 = Build Array(w478, w475, 0.0 ("element"), 0.0 ("element")) -> (w456:dbl[])
        n156 = Add(x=w456, y=w476) -> (x+y=w443:dbl[])
        n157 = Add(x=w444, y=w443) -> (x+y=w462:dbl[])
        "Needle parking position" <- w462
        n158 = call "XYZTheta Go.vi"("XYZTheta In"=w462, "Motion in"=w463) -> ("error out"=w474:errorcluster, "XYZTheta Out"=w472:dbl[], "Motion out"=w461:refnum<class "Motion.lvclass">)  [unwired: 7 in]
        n159 = call "Display Message to User"("error in (no error)"=w474) -> ("error out"=w464:errorcluster)  [unwired: 9 in, 1 out]
        n160 = Select(t=dbl[][] [[-8.43, -62.0, 4.0, 4.0], [-5.62, -59.0, 4.0, 4.0], [-2.81, -56.0, 4.0, 4.0], [0.0, -53.0, 1.0, 1.0], [-8.43, -48.0, 4.0, 0.0], [-5.62, -45.0, 4.0, 0.0], [-2.81, -42.0, 4.0, 0.0], [0.0, -39.0, 1.0, 0.0]], s=w438, f=dbl[][] [[-8.43, -48.0, 4.0, 4.0], [-5.62, -45.0, 4.0, 4.0], [-2.81, -42.0, 4.0, 4.0], [0.0, -39.0, 1.0, 1.0], [-8.43, -62.0, 4.0, 0.0], [-5.62, -59.0, 4.0, 0.0], [-2.81, -56.0, 4.0, 0.0], [0.0, -53.0, 1.0, 0.0]]) -> (s? t:f=w435:dbl[][])
        n161 = Index Array(array=w472, index=2) -> (element=w468:dbl)
        n162 = call-dynamic "Z Go.vi"("error in (no error)"=w464, "Speed"=20.0, "Position"=0.0, "Motion in"=w461) -> ("error out"=w460:errorcluster, "Motion out"=w467:refnum<class "Motion.lvclass">)  [unwired: 6 in]
        n163 = call "Display Message to User2"("error in (no error)"=w460) -> ("error out"=w459:errorcluster)  [unwired: 9 in, 1 out]
        n164 = Add(x=w468, y=-2.5) -> (x+y=w469:dbl)
        n165 = call-dynamic "Z Go.vi"("error in (no error)"=w459, "Speed"=20.0, "Position"=w469, "Motion in"=w467) -> ("error out"=w457:errorcluster, "Motion out"=w458:refnum<class "Motion.lvclass">)  [unwired: 6 in]
        n166 = call-dynamic "Connect.vi"("Ultimus V in"=refnum<class "Ultimus V2.lvclass"> refnum ("Ultimus V2.lvclass")) -> ("Ultimus V out"=w455:refnum<class "Ultimus V2.lvclass">)  [unwired: 9 in, 1 out]
        n167 = case shown="True" w447 {
          tunnel: w458 -> [w498 w609]
          tunnel: w457 -> [w499 w608]
          tunnel: [w497 w607] -> w452
          tunnel: [w499 w606] -> w450
          tunnel: w446 -> [w494 w600]
          tunnel: w456 -> [w493 w605]
          tunnel: w455 -> [w495 w604]
          tunnel: [w496 w603] -> w453
          tunnel: w445 -> [w492 w602]
          tunnel: w435 -> [w491 _]
          tunnel: "Needle Height Compenstation\n(glue gap)" -> [w490 w601]
          tunnel: "check height?" -> [w489 w598]
          frame False {
            # "two sensor, Sensor B then A"
            n168 = for {
              N: w492 -> [_]
              tunnel: w498 -> [w515]
              tunnel: [w514] -> w496
              tunnel: [w513] -> w497
              tunnel: w495 -> [w512]
              tunnel: w494 -> [w511] mode=indexing
              tunnel: w493 -> [w505]
              tunnel: w491 -> [w507]
              tunnel: w490 -> [w501]
              tunnel: w489 -> [w500]
              i -> [w503]
              # "four\nloops"
              n169 = Multiply(x=4, y=w503) -> (x*y=w502:i32)
              n170 = Array Subset(array=w507, index (row)=w502, length (row)=4 ("length"), index (col)=0, length (col)=3 ("length")) -> (w506:dbl[][])
              "GlueBox" <- w506
              n171 = for {
                N: 4 -> [_]
                tunnel: w515 -> [w577]
                tunnel: [w569] -> w514
                tunnel: [w564] -> w513
                tunnel: w512 -> [w556]
                tunnel: w511 -> [w534]
                tunnel: w506 -> [w531] mode=indexing
                tunnel: w505 -> [w537]
                tunnel: w501 -> [w523]
                tunnel: w500 -> [w520]
                n172 = Index Array(array=w531, index=0) -> (element=w553:dbl)
                n173 = Index Array(array=w531, index=1) -> (element=w552:dbl)
                n174 = Array Subset(array=w534, index=0, length=2) -> (w536:dbl[])
                n175 = Add(x=w536, y=w537) -> (x+y=w535:dbl[])
                n176 = Absolute Value(x=w553) -> (abs(x)=w551:dbl)
                n177 = Absolute Value(x=w552) -> (abs(x)=w549:dbl)
                n178 = Add(x=w535, y=w531) -> (x+y=w546:dbl[])
                n179 = Multiply(x=w549, y=2.0) -> (x*y=w527:dbl)
                n180 = Multiply(x=w551, y=2.0) -> (x*y=w528:dbl)
                n181 = Multiply(x=w527, y=-1.0) -> (x*y=w539:dbl)
                n182 = Build Array(0.0 ("element"), w527) -> (w547:dbl[])
                n183 = Build Array(w528, 0.0 ("element")) -> (w544:dbl[])
                n184 = Build Array(0.0 ("element"), w539) -> (w525:dbl[])
                n185 = Add(x=w546, y=w547) -> (x+y=w543:dbl[])
                n186 = Add(x=w543, y=w544) -> (x+y=w526:dbl[])
                n187 = call-dynamic "XY Go.vi"("Speed"=200.0, "XY"=w546, "Motion in"=w577) -> ("error out"=w529:errorcluster, "Motion out"=w576:refnum<class "Motion.lvclass">)  [unwired: 7 in]
                n188 = Add(x=w526, y=w525) -> (x+y=w524:dbl[])
                n189 = Index Array(array=w534, index=2) -> (element=w533:dbl)
                n190 = Index Array(array=w531, index=2) -> (element=w530:dbl)
                n191 = Add(x=w533, y=w523) -> (x+y=w562:dbl)
                n192 = Build Array(w543, w526, w524, w546) -> (w538:dbl[][])
                "appended array" <- w538
                n193 = call-dynamic "Z Go.vi"("error in (no error)"=w529, "Speed"=5.0, "Position"=w562, "Motion in"=w576) -> ("error out"=w522:errorcluster, "Motion out"=w572:refnum<class "Motion.lvclass">)  [unwired: 6 in]
                n194 = case shown="True" w520 {
                  tunnel: w522 -> [w589 w591]
                  tunnel: [w589 w590] -> w521
                  frame False {
                  }
                  frame True {
                    n195 = call "Display Message to User11"("error in (no error)"=w591) -> ("error out"=w590:errorcluster)  [unwired: 9 in, 1 out]
                  }
                }
                n196 = call "vacuum.vi"("error in (no error)"=w521, "Vacuum Setting (0000)"=i64 100, "Ultimus V in"=w556) -> ("error out"=w574:errorcluster, "Ultimus V out"=w559:refnum<class "Ultimus V2.lvclass">)  [unwired: 7 in]
                n197 = flat-sequence {
                  tunnel: w559 -> [w582]
                  tunnel: w574 -> [w583]
                  tunnel: [w583] -> w519
                  tunnel: [w582] -> w518
                  tunnel: [w581] -> w517
                  tunnel: [w588] -> w575
                  tunnel: [w585] -> w558
                  tunnel: w519 -> [w587]
                  tunnel: w518 -> [w586]
                  tunnel: w517 -> [w584]
                  frame #0 {
                    n198 = call "air pressure setting.vi"() -> ("air pressure indecator"=w581:i32)  [unwired: 1 out]
                  }
                  frame #1 {
                    n199 = call-dynamic "Pressure.vi"("error in (no error)"=w587, "Pressure"=w584, "Ultimus V in"=w586) -> ("error out"=w588:errorcluster, "Ultimus V out"=w585:refnum<class "Ultimus V2.lvclass">)  [unwired: 7 in]
                  }
                }
                n200 = call-dynamic "Dispense.vi"("error in (no error)"=w575, "Ultimus V in"=w558) -> ("error out"=w571:errorcluster, "Ultimus V out"=w557:refnum<class "Ultimus V2.lvclass">)  [unwired: 8 in]
                n201 = for {
                  N: w530 -> [_]
                  tunnel: w572 -> [w597]
                  tunnel: w571 -> [w596]
                  tunnel: [w595] -> w570
                  tunnel: [w594] -> w568
                  tunnel: w538 -> [w593] mode=indexing
                  (unwired) 4.5 ("Speed")
                  n202 = call-dynamic "XY Go.vi"("error in (no error)"=w596, "Speed"=4.5, "XY"=w593, "Motion in"=w597) -> ("error out"=w595:errorcluster, "Motion out"=w594:refnum<class "Motion.lvclass">)  [unwired: 6 in]
                }
                n203 = Add(x=w562, y=-2.0) -> (x+y=w565:dbl)
                n204 = call-dynamic "Dispense.vi"("error in (no error)"=w570, "Ultimus V in"=w557) -> ("error out"=w563:errorcluster, "Ultimus V out"=w569:refnum<class "Ultimus V2.lvclass">)  [unwired: 8 in]
                n205 = call-dynamic "Z Go.vi"("error in (no error)"=w563, "Speed"=10.0, "Position"=w565, "Motion in"=w568) -> ("Motion out"=w564:refnum<class "Motion.lvclass">)  [unwired: 6 in, 1 out]
              }
            }
          }
          frame True {
            n206 = case shown="True" w598 {
              tunnel: w600 -> [w610 w614]
              tunnel: [w610 w611] -> w599
              frame False {
              }
              frame True {
                n207 = Array Subset(array=w614, index (row)=12 ("index"), length (row)=4 ("length")) -> (w611:dbl[][])  [unwired: 2 in]
              }
            }
            n208 = for {
              N: w602 -> [_]
              tunnel: w609 -> [w654]
              tunnel: w608 -> [w653]
              tunnel: [w639] -> w603
              tunnel: [w638] -> w607
              tunnel: [w637] -> w606
              tunnel: w599 -> [w625] mode=indexing
              tunnel: w605 -> [w624]
              tunnel: w604 -> [w623]
              tunnel: w601 -> [w621]
              tunnel: w598 -> [w618]
              # "move the glue in x-dir\n0.1 mm closer to center"
              n209 = Index Array(array=w625, index=2) -> (element=w626:dbl)
              n210 = Add(x=w625, y=w624) -> (x+y=w652:dbl[])
              n211 = Build Array(0.0 ("element"), 3.3 ("element")) -> (w657:dbl[])
              n212 = Subtract(x=w652, y=w657) -> (x-y=w658:dbl[])
              n213 = Add(x=w626, y=w621) -> (x+y=w627:dbl)
              n214 = Add(x=w652, y=w657) -> (x+y=w635:dbl[])
              n215 = call-dynamic "XY Go.vi"("error in (no error)"=w653, "Speed"=200.0, "XY"=w658, "Motion in"=w654) -> ("error out"=w640:errorcluster, "Motion out"=w633:refnum<class "Motion.lvclass">)  [unwired: 6 in]
              n216 = call-dynamic "Z Go.vi"("error in (no error)"=w640, "Speed"=5.0, "Position"=w627, "Motion in"=w633) -> ("error out"=w620:errorcluster)  [unwired: 6 in, 1 out]
              n217 = case shown="True" w618 {
                tunnel: w620 -> [w667 w669]
                tunnel: [w667 w668] -> w619
                frame False {
                }
                frame True {
                  n218 = call "Display Message to User7"("error in (no error)"=w669) -> ("error out"=w668:errorcluster)  [unwired: 9 in, 1 out]
                }
              }
              n219 = call "vacuum.vi"("error in (no error)"=w619, "Vacuum Setting (0000)"=i64 100, "Ultimus V in"=w623) -> ("error out"=w649:errorcluster, "Ultimus V out"=w644:refnum<class "Ultimus V2.lvclass">)  [unwired: 7 in]
              n220 = flat-sequence {
                tunnel: w644 -> [w660]
                tunnel: w649 -> [w661]
                tunnel: [w661] -> w617
                tunnel: [w660] -> w616
                tunnel: [w659] -> w615
                tunnel: [w666] -> w650
                tunnel: [w663] -> w642
                tunnel: w617 -> [w665]
                tunnel: w616 -> [w664]
                tunnel: w615 -> [w662]
                frame #0 {
                  n221 = call "air pressure setting.vi"() -> ("air pressure indecator"=w659:i32)  [unwired: 1 out]
                }
                frame #1 {
                  n222 = call-dynamic "Pressure.vi"("error in (no error)"=w665, "Pressure"=w662, "Ultimus V in"=w664) -> ("error out"=w666:errorcluster, "Ultimus V out"=w663:refnum<class "Ultimus V2.lvclass">)  [unwired: 7 in]
                }
              }
              n223 = call-dynamic "Dispense.vi"("error in (no error)"=w650, "Ultimus V in"=w642) -> ("error out"=w634:errorcluster, "Ultimus V out"=w641:refnum<class "Ultimus V2.lvclass">)  [unwired: 8 in]
              n224 = call "Time Delay"("error in (no error)"=w634) -> ("error out"=w632:errorcluster)  [unwired: 10 in]
              n225 = call-dynamic "XY Go.vi"("error in (no error)"=w632, "Speed"=5.0, "XY"=w635, "Motion in"=w633) -> ("error out"=w631:errorcluster, "Motion out"=w629:refnum<class "Motion.lvclass">)  [unwired: 6 in]
              n226 = call "Time Delay3"("error in (no error)"=w631) -> ("error out"=w630:errorcluster)  [unwired: 10 in]
              n227 = call "Time Delay2"("error in (no error)"=w632) -> ("error out"=w643:errorcluster)  [unwired: 10 in]
              n228 = call-dynamic "Dispense.vi"("error in (no error)"=w643, "Ultimus V in"=w641) -> ("Ultimus V out"=w639:refnum<class "Ultimus V2.lvclass">)  [unwired: 8 in, 1 out]
              n229 = Add(x=w627, y=-2.5) -> (x+y=w647:dbl)
              n230 = call-dynamic "Z Go.vi"("error in (no error)"=w630, "Speed"=10.0, "Position"=w647, "Motion in"=w629) -> ("error out"=w637:errorcluster, "Motion out"=w638:refnum<class "Motion.lvclass">)  [unwired: 6 in]
            }
          }
        }
        n231 = call-dynamic "Disconnect.vi"("Ultimus V in"=w453) -> ()  [unwired: 9 in, 1 out]
        n232 = call "XYZTheta Go.vi"("error in (no error)"=w450, "XYZTheta In"=dbl[] [400.0, 625.0, 0.0, 0.1], "Motion in"=w452) -> ("error out"=w451:errorcluster, "Motion out"=w448:refnum<class "Motion.lvclass">)  [unwired: 6 in, 1 out]
        n233 = call "Display Message to User3"("error in (no error)"=w451) -> ()  [unwired: 9 in, 2 out]
      }
      event "Needle Alignment": Value Change {
        (unwired) "Needle Alignment in progress ...." ("String")
        # "first needle park position\nneedle gap on Z value : 0.5 mm"
        # "Syringe-camera offset"
        n234 = event-data() -> ()  [unwired: 1 in, 6 out]
        n235 = call-poly <vilib>:"Read Delimited Spreadsheet.vi"("file path (dialog if empty)"=path "D:/INTT/V1/Assembly Data/Tool Offsets/Dispense Tip Offset.txt", "number of rows (all:-1)"=-1) -> ("first row"=w712:dbl[])  [unwired: 8 in, 5 out]
        n236 = Build Array(11.75, -25, 0.5 ("element"), 0.0 ("element")) -> (w705:dbl[])
        n237 = Index Array(array=w712, index #1=0 ("index"), index #2=1 ("index")) -> (element #1=w707:dbl, element #2=w704:dbl)
        n238 = Build Array(w707, w704, 0.0 ("element"), 0.0 ("element")) -> (w674:dbl[])
        n239 = Add(x=w674, y=w705) -> (x+y=w698:dbl[])
        n240 = Add(x=w697, y=w698) -> (x+y=w699:dbl[])
        n241 = call "XYZTheta Go.vi"("XYZTheta In"=w699, "Motion in"=w689) -> ("error out"=w703:errorcluster, "XYZTheta Out"=w679:dbl[], "Motion out"=w688:refnum<class "Motion.lvclass">)  [unwired: 7 in]
        n242 = call "Display Message to User10"("error in (no error)"=w703) -> ("error out"=w700:errorcluster)  [unwired: 9 in, 1 out]
        n243 = call-dynamic "Z Go.vi"("error in (no error)"=w700, "Speed"=20.0, "Position"=0.0, "Motion in"=w688) -> ("Motion out"=w687:refnum<class "Motion.lvclass">)  [unwired: 6 in, 1 out]
        n244 = Replace Array Subset(array=w679, new element=0.0 ("new element/subarray"), index=2) -> (w676:dbl[])
        n245 = call "Joystick and Camera SHIH VPC- external Connection.vi"("Motion in"=w687, "XYZTheta"=w676, "Measurement Point"="Touch Needle on a surface") -> ("Motion out"=w685:refnum<class "Motion.lvclass">, "Gantry"=w675:dbl[])  [unwired: 4 in, 2 out]
        n246 = Subtract(x=w675, y=w674) -> (x-y=w673:dbl[])
        n247 = call "Joystick and Camera SHIH VPC- external Connection.vi"("Motion in"=w685, "XYZTheta"=w673, "Measurement Point"="Measure the touch spot with camera") -> ("Motion out"=w681:refnum<class "Motion.lvclass">, "Gantry"=w684:dbl[])  [unwired: 4 in, 2 out]
        n248 = Subtract(x=w675, y=w684) -> (x-y=w683:dbl[])
        n249 = call-poly <vilib>:"Write Delimited Spreadsheet.vi"("file path (dialog if empty)"=path "D:/INTT/V1/Assembly Data/Tool Offsets/Dispense Tip Offset.txt", "1D data"=w683, "append to file? (new file:F)"=FALSE) -> ()  [unwired: 11 in, 2 out]
      }
      event "Pick and place": Value Change {
        (unwired) "PICK and PLACE samples ..." ("String")
        (unwired) -21.3804 ("new element/subarray")
        n250 = event-data() -> ()  [unwired: 1 in, 6 out]
        n251 = call-poly <vilib>:"Read Delimited Spreadsheet.vi"("file path (dialog if empty)"=path "D:/INTT/V1/Assembly Data/Tool Offsets/Bellows Tool Offset.txt", "number of rows (all:-1)"=-1) -> ("first row"=w743:dbl[])  [unwired: 8 in, 5 out]
        n252 = Select(t=1, s=w720, f=w732) -> (s? t:f=w748:i32)
        n253 = Index Array(array=w743, index #1=0 ("index"), index #2=1 ("index"), index #3=2 ("index")) -> (element #1=w739:dbl, element #2=w738:dbl, element #3=w737:dbl)
        n254 = case shown="True" w728 {
          tunnel: [w749 w752] -> w727
          tunnel: w722 -> [w749 w751]
          frame False {
          }
          frame True {
            # "sensor A"
            # "sensor B"
            n255 = Index Array(array=w751, index=0) -> (element=w750:i32)
            n256 = Index Array(array=w751, index=1) -> (element=w753:i32)
            n257 = Build Array(w753, w750) -> (w752:i32[])
          }
        }
        n258 = for {
          N: w748 -> [_]
          tunnel: w732 -> [w792]
          tunnel: w733 -> [w788]
          tunnel: w746 -> [w812]
          tunnel: [w800] -> w736
          tunnel: w734 -> [w810] mode=indexing
          tunnel: [w776] -> w726
          tunnel: w725 -> [w764]
          tunnel: w739 -> [w802]
          tunnel: w738 -> [w801]
          tunnel: w735 -> [w785]
          tunnel: w737 -> [w799]
          tunnel: w720 -> [w769]
          tunnel: w727 -> [w758] mode=indexing
          tunnel: "VacChannel for sample" -> [w771]
          tunnel: "check height? 2" -> [w756]
          tunnel: w720 -> [w757]
          i -> [w778]
          w762 = 0 ("Channel")
          w761 = TRUE ("Value")
          # "put back pickup tool"
          # "if chips, do one pickup tool and multiple samples;\nif sensors, one pickup tool for one sample ( so 2->2);"
          # "build a fake 2d arrays"
          # "sensor"
          # "chip pickup tool"
          # "pickup tool height offset"
          # "Pick up PICKUP TOOL"
          # "Pick up CHIPs/Sensor and place on HDI"
          n259 = Select(t=w792, s=w769, f=1) -> (s? t:f=w791:i32)
          n260 = Build Array(w802, w801, w799, 0.0 ("element")) -> (w797:dbl[])
          n261 = Add(x=w810, y=w797) -> (x+y=w798:dbl[])
          n262 = call "XYZTheta-2Zspeed Go.vi"("XYZTheta In"=w798, "Motion in"=w812) -> ("error out"=w760:errorcluster, "Motion out"=w811:refnum<class "Motion.lvclass">)  [unwired: 7 in, 1 out]
          n263 = Select(t=-18.52 ("new element/subarray"), s=w769, f=-13.13 ("t")) -> (s? t:f=w793:dbl)
          n264 = call "WriteReadWait.vi"("Read Value"=w761, "Write Value"=w761, "error in (no error)"=w760, "Read"=w762, "Write"=w762, "I-O in"=w764) -> ("error out"=w759:errorcluster, "I-O out"=w763:refnum<class "NI-DAQ.lvclass">)  [unwired: 4 in]
          n265 = Replace Array Subset(array=w797, new element=w793, index=2) -> (w795:dbl[])
          n266 = Index Array(array=w788, index (row)=w778) -> (element=w787:dbl[])  [unwired: 1 in]
          n267 = call "Time Delay8"("error in (no error)"=w759) -> ("error out"=w808:errorcluster)  [unwired: 10 in]
          n268 = Build Array(w787, w787) -> (w786:dbl[][])
          n269 = Select(t=w788, s=w769, f=w786) -> (s? t:f=w789:dbl[][])
          n270 = Index Array(array=w785, index (row)=w778) -> (element=w784:dbl[])  [unwired: 1 in]
          n271 = Build Array(w784, w784) -> (w783:dbl[][])
          n272 = Select(t=w785, s=w769, f=w783) -> (s? t:f=w766:dbl[][])
          n273 = case shown="False" w756 {
            tunnel: [w813 w815] -> w765
            tunnel: w766 -> [w813 w814]
            frame False {
            }
            frame True {
              n274 = Array Subset(array=w814, index (row)=12 ("index"), length (row)=4 ("length")) -> (w815:dbl[][])  [unwired: 2 in]
            }
          }
          n275 = Select(t="chip placement height compensation", s=w769, f=0.0) -> (s? t:f=w767:dbl)
          n276 = for {
            N: w791 -> [_]
            tunnel: w789 -> [w832] mode=indexing
            tunnel: w811 -> [w834]
            tunnel: w795 -> [w833]
            tunnel: w808 -> [w831]
            tunnel: [w830] -> w803
            tunnel: w763 -> [w829]
            tunnel: w765 -> [w826] mode=indexing
            tunnel: [w825] -> w794
            tunnel: w767 -> [w824]
            tunnel: w758 -> [w823]
            tunnel: w771 -> [w822]
            tunnel: [w821] -> w770
            tunnel: w769 -> [w820]
            tunnel: w756 -> [w819]
            tunnel: w757 -> [w818]
            n277 = flat-sequence {
              tunnel: w832 -> [w851]
              tunnel: [w853] -> w835
              tunnel: w834 -> [w852]
              tunnel: w833 -> [w850]
              tunnel: w831 -> [w848]
              tunnel: w829 -> [w846]
              tunnel: [w840] -> w828
              tunnel: [w841] -> w827
              tunnel: w823 -> [w843]
              tunnel: w822 -> [w838]
              tunnel: w835 -> [w879]
              tunnel: [w878] -> w830
              tunnel: w833 -> [w876]
              tunnel: w828 -> [w877]
              tunnel: w827 -> [w864]
              tunnel: w826 -> [w875]
              tunnel: [w854] -> w825
              tunnel: w824 -> [w868]
              tunnel: w822 -> [w863]
              tunnel: [w859] -> w821
              tunnel: w820 -> [_]
              tunnel: w819 -> [w865]
              tunnel: w818 -> [w858]
              frame #0 {
                w839 = TRUE ("Value")
                w842 = FALSE ("Value")
                # "pickup sample"
                # "release sample from tray"
                # "pickup sample from tray"
                n278 = Add(x=w851, y=w850) -> (x+y=w849:dbl[])
                n279 = call "XYZTheta-2Zspeed Go.vi"("error in (no error)"=w848, "XYZTheta In"=w849, "Motion in"=w852) -> ("error out"=w847:errorcluster, "Motion out"=w853:refnum<class "Motion.lvclass">)  [unwired: 6 in, 1 out]
                n280 = call "Time Delay4"("error in (no error)"=w847) -> ("error out"=w844:errorcluster)  [unwired: 10 in]
                n281 = call "WriteReadWait.vi"("Read Value"=w842, "Write Value"=w842, "error in (no error)"=w844, "Read"=w843, "Write"=w843, "I-O in"=w846) -> ("error out"=w845:errorcluster, "I-O out"=w837:refnum<class "NI-DAQ.lvclass">)  [unwired: 4 in]
                n282 = call "Time Delay11"("error in (no error)"=w845) -> ("error out"=w836:errorcluster)  [unwired: 10 in]
                n283 = call "WriteReadWait.vi"("Read Value"=w839, "Write Value"=w839, "error in (no error)"=w836, "Read"=w838, "Write"=w838, "I-O in"=w837) -> ("error out"=w840:errorcluster, "I-O out"=w841:refnum<class "NI-DAQ.lvclass">)  [unwired: 4 in]
              }
              frame #1 {
                w861 = FALSE ("Value")
                # "release sample on HDI"
                # "lift for chip/sensor thickness"
                # "place sample on HDI"
                n284 = Add(x=w875, y=w876) -> (x+y=w871:dbl[])
                n285 = Build Array(0.0 ("element"), 0.0 ("element"), w868, 0.0 ("element")) -> (w870:dbl[])
                n286 = Add(x=w871, y=w870) -> (x+y=w869:dbl[])
                n287 = call "XYZTheta-2Zspeed Go.vi"("error in (no error)"=w877, "XYZTheta In"=w869, "Motion in"=w879) -> ("error out"=w867:errorcluster, "Motion out"=w878:refnum<class "Motion.lvclass">)  [unwired: 6 in, 1 out]
                n288 = case shown="False" w865 {
                  tunnel: w867 -> [w885 w887]
                  tunnel: [w885 w886] -> w866
                  frame False {
                  }
                  frame True {
                    n289 = call "Display Message to User6"("error in (no error)"=w887) -> ("error out"=w886:errorcluster)  [unwired: 9 in, 1 out]
                  }
                }
                n290 = case shown="False" w858 {
                  tunnel: w866 -> [w882 w884]
                  tunnel: [w880 w883] -> w862
                  frame False {
                    n291 = call "Time Delay7"("error in (no error)"=w882) -> ("error out"=w881:errorcluster)  [unwired: 10 in]
                    n292 = call "ser8"("error in (no error)"=w881) -> ("error out"=w880:errorcluster)  [unwired: 9 in, 1 out]
                  }
                  frame True {
                    n293 = call "Time Delay6"("error in (no error)"=w884) -> ("error out"=w883:errorcluster)  [unwired: 10 in]
                  }
                }
                n294 = call "WriteReadWait.vi"("Read Value"=w861, "Write Value"=w861, "error in (no error)"=w862, "Read"=w863, "Write"=w863, "I-O in"=w864) -> ("error out"=w860:errorcluster, "I-O out"=w859:refnum<class "NI-DAQ.lvclass">)  [unwired: 4 in]
                n295 = call "Time Delay5"("error in (no error)"=w860) -> ("error out"=w857:errorcluster)  [unwired: 10 in]
                n296 = call "message 10"("error in (no error)"=w857) -> ("error out"=w856:errorcluster)  [unwired: 9 in, 1 out]
                n297 = call "Time Delay12"("error in (no error)"=w856) -> ("error out"=w855:errorcluster)  [unwired: 10 in]
                n298 = call "message 9"("error in (no error)"=w855) -> ("error out"=w854:errorcluster)  [unwired: 9 in, 1 out]
              }
            }
          }
          n299 = call "XYZTheta-2Zspeed Go.vi"("error in (no error)"=w794, "XYZTheta In"=w798, "Motion in"=w803) -> ("error out"=w768:errorcluster, "Motion out"=w807:refnum<class "Motion.lvclass">)  [unwired: 6 in, 1 out]
          n300 = call "Time Delay9"("error in (no error)"=w768) -> ("error out"=w774:errorcluster)  [unwired: 10 in]
          n301 = call-dynamic "Digital Write 1 Channel.vi"("DAQ Module"=0, "error constant"=w774, "Value"=FALSE, "Channel"=0, "NI-DAQ.lvclass"=w770) -> ("error IO"=w777:errorcluster, "NI-DAQ.lvclass 2"=w776:refnum<class "NI-DAQ.lvclass">)  [unwired: 5 in]
          n302 = call "Time Delay10"("error in (no error)"=w777) -> ("error out"=w804:errorcluster)  [unwired: 10 in]
          n303 = call-dynamic "Z Go.vi"("error in (no error)"=w804, "Speed"=20.0, "Position"=0.0 ("new element/subarray"), "Motion in"=w807) -> ("Motion out"=w800:refnum<class "Motion.lvclass">)  [unwired: 6 in, 1 out]
        }
      }
      event "GOTO": Value Change {
        (unwired) "GOING to a position" ("String")
        n304 = event-data() -> ()  [unwired: 1 in, 6 out]
        n305 = call "XYZTheta-2Zspeed Go.vi"("XYZTheta In"="Parking position", "Motion in"=w892) -> ("Motion out"=w891:refnum<class "Motion.lvclass">)  [unwired: 7 in, 2 out]
      }
      event "READ Position": Value Change {
        n306 = event-data() -> ()  [unwired: 1 in, 6 out]
        n307 = call-dynamic "Get Current Position.vi"("Motion in"=w915) -> ("XYZTheta Out"=→"Gantry current position":dbl[], "Motion out"=w914:refnum<class "Motion.lvclass">)  [unwired: 8 in, 1 out]
      }
      event "TrayVaccum": Value Change {
        n308 = event-data() -> ()  [unwired: 1 in, 6 out]
        n309 = Index Array(array=w919, index=0) -> (element=w928:i32)
        n310 = Index Array(array="Values", index=0) -> (element=w922:bool)
        n311 = call "WriteReadWait.vi"("Read Value"=w922, "Write Value"=w922, "Read"=w928, "Write"=w928, "I-O in"=w931) -> ("error out"=w927:errorcluster, "I-O out"=w930:refnum<class "NI-DAQ.lvclass">)  [unwired: 5 in]
        n312 = Index Array(array=w919, index=1) -> (element=w925:i32)
        n313 = Index Array(array="Values", index=1) -> (element=w920:bool)
        n314 = call "WriteReadWait.vi"("Read Value"=w920, "Write Value"=w920, "error in (no error)"=w927, "Read"=w925, "Write"=w925, "I-O in"=w930) -> ("I-O out"=w917:refnum<class "NI-DAQ.lvclass">)  [unwired: 4 in, 1 out]
      }
      event Timeout {
        n315 = event-data() -> ()  [unwired: 1 in, 3 out]
        n316 = call-dynamic "Digital Read Multiple Channels.vi"("Array"=w946, "NI-DAQ in"=w945) -> ("subarray"=w947:bool[], "NI-DAQ out"=w943:refnum<class "NI-DAQ.lvclass">)  [unwired: 7 in, 1 out]
      }
    }
    "Measure HDI top-left" <- w42
    "Sample on HDI" <- w14
    "vacuum on?" <- w18
    "Sample on HDI aspect to drawing" <- w13
    n317 = feedback-in #1(w40) -> ()
    n318 = feedback-in #2(w42) -> ()
    n319 = feedback-in #3(w37) -> ()
    n320 = feedback-in #4(w29) -> ()
    n321 = feedback-in #5(w26) -> ()
    n322 = feedback-in #6(w18) -> ()
    n323 = feedback-in #7(w34) -> ()
    n324 = feedback-in #9(w13) -> ()
    n325 = feedback-in #10(w35) -> ()
    "# of tasks excuted" <- w31
  }
  n326 = call-dynamic "Disconnect.vi"("I-O in"=w1) -> ()  [unwired: 9 in, 1 out]
  n327 = call-dynamic "Disconnect.vi"("Controller in"=w4) -> ()  [unwired: 9 in, 1 out]
